vi "Modified RTS CTS.vi"() -> ()   [LabVIEW 2012]
uses:
  <vilib>/measure/maspectr.llb/FFT Power Spectrum and PSD for 1 Chan.vi
  <instrlib>/niUSRP/niUSRP Fetch Rx Data (CDB Cluster).vi
  <vilib>/addons/Modulation/Digital/General/MT Map Bits to QAM Symbols.vi
  <instrlib>/niUSRP/niUSRP Write Tx Data (CDB).vi
  <vilib>/Analysis/2dsp.llb/Inverse Complex FFT.vi
  <instrlib>/niUSRP/niUSRP Fetch Rx Data (CDB).vi
  <vilib>/Analysis/2dsp.llb/Complex FFT.vi
  <vilib>/addons/Modulation/Digital/General/MT Map QAM Symbols to Bits.vi
  <vilib>/addons/Modulation/Digital/General/MT Generate PSK System Parameters(M).vi
  <instrlib>/niUSRP/niUSRP Write Tx Data (CDB Cluster).vi
  <vilib>/Analysis/NI_AALPro.lvlib
  <vilib>/addons/Modulation/niDMT.lvlib
  <vilib>/measure/NI_MAPro.lvlib
panel:
  in  "stop 2":bool
  out "String":string
  in  "millisecond multiple":u32
  out "millisecond timer value 5":u32
  out "Enter control signal (1,2 or 3)\n1. Power\n2. Trade Off\n3. Bandwidth 2":string
  out "Symbol Rate\n[symbols/sec]":dbl=25000.0 format="%#.6p"
  in  "BPSK System Parameters 9":T1={"Samples per Symbol"=8, "symbol map"=[], "Differential PSK"=enum."disable", "PSK type"=0} caption="BPSK System Parameters" {"PSK type" items=["normal", "shifted", "offset"]; "symbol map" format="%.3f"}
  in  "BPSK System Parameters 8":T1={"Samples per Symbol"=8, "symbol map"=[], "Differential PSK"=enum."disable", "PSK type"=0} caption="BPSK System Parameters" {"PSK type" items=["normal", "shifted", "offset"]; "symbol map" format="%.3f"}
  in  "BPSK System Parameters 7":T1={"Samples per Symbol"=8, "symbol map"=[], "Differential PSK"=enum."disable", "PSK type"=0} caption="BPSK System Parameters" {"PSK type" items=["normal", "shifted", "offset"]; "symbol map" format="%.3f"}
  in  "BPSK System Parameters 6":T1={"Samples per Symbol"=8, "symbol map"=[], "Differential PSK"=enum."disable", "PSK type"=0} caption="BPSK System Parameters" {"PSK type" items=["normal", "shifted", "offset"]; "symbol map" format="%.3f"}
  in  "BPSK System Parameters 5":T1={"Samples per Symbol"=8, "symbol map"=[], "Differential PSK"=enum."disable", "PSK type"=0} caption="BPSK System Parameters" {"PSK type" items=["normal", "shifted", "offset"]; "symbol map" format="%.3f"}
  in  "BPSK System Parameters 4":T1={"Samples per Symbol"=8, "symbol map"=[], "Differential PSK"=enum."disable", "PSK type"=0} caption="BPSK System Parameters" {"PSK type" items=["normal", "shifted", "offset"]; "symbol map" format="%.3f"}
  in  "BPSK System Parameters 3":T1={"Samples per Symbol"=8, "symbol map"=[], "Differential PSK"=enum."disable", "PSK type"=0} caption="BPSK System Parameters" {"PSK type" items=["normal", "shifted", "offset"]; "symbol map" format="%.3f"}
  in  "Tab Control 3":T2(tab)
  in  "Enter control signal (1,2 or 3)\n1. Power\n2. Trade Off\n3. Bandwidth":string
  in  "Packet Parameters":T3={"Guard Bits "=30, "Sync Bits"=20, "Message Bits"=128}
  in  "Packet Pad \n[samples]":i32=200
  in  "Blank Frame \n[samples]":i32=500
  out "Number of Packets in Message":i32=46
  in  "PN sequence order\nfor Sync Bits":i32=31 caption="PN sequence order (9)"
  in  "Packet Repeat":i32=2
  in  "Pulse Shaping Filter Parameters":T4={"Alpha"=0.5, "Filter Length"=6, "TX Filter"=enum."Root Raised Cos"} caption="Pulse Shaping Filter" {"Alpha" format="%.2f"}
  in  "Tx Parameters":T5={"Tx IQ Sampling\nRate [s/sec]"=500000.0, "Tx Frequency [Hz]"=2500000000.0, "Tx Gain [dB]"=0.0, "Tx Antenna"="TX1"} {"Tx Gain [dB]" format="%#.6p"; "Tx Frequency [Hz]" format="%#.6p"; "Tx IQ Sampling\nRate [s/sec]" format="%#.6p"}
  out "Actual Tx Parameters":T5={"Tx IQ Sampling\nRate [s/sec]"=200000.0, "Tx Frequency [Hz]"=2500000000.0, "Tx Gain [dB]"=0.0, "Tx Antenna"="TX1"} {"Tx Gain [dB]" format="%#.6p"; "Tx Frequency [Hz]" format="%#.6p"; "Tx IQ Sampling\nRate [s/sec]" format="%#.6p"}
  in  "USRP IP address":refnum<k15>="192.168.10.2"
  out "error out 4":errorcluster
  in  "Queue Length":i32=10
  in  "stop":bool
  out "result":bool
  out "Constellation Graph":T6(graph)
  in  "autoscale":bool
  in  "millisecond multiple 2":u32
  out "millisecond timer value 4":u32
  out "x = y?":bool
  out "Boolean":bool
  out "Message Text 3":string="Two roads diverged in a yellow wood,\nAnd sorry I could not travel both\nAnd be one traveler, long I stood\nAnd looked down one as far as I could\nTo where it bent in the undergrowth.\n\nThen took the other, as just as fair,\nAnd having perhaps the better claim,\nBecause it was grassy and wanted wear;\nThough as for that the passing there\nHad worn them really about the same.\n\nAnd both that morning equally lay\nIn leaves no step had trodden black.\nOh, I kept the first for another day!\nYet knowing how way leads on to way,\nI doubted if I should ever come back.\n\nI shall be telling this with a sigh\nSomewhere ages and ages hence:\nTwo roads diverged in a wood, and I--\nI took the one less traveled by,\nAnd that has made all the difference.\n"
  out "M-PSK (4)":i32
  in  "Tx Parameters 3":T5={"Tx IQ Sampling\nRate [s/sec]"=500000.0, "Tx Frequency [Hz]"=2500000000.0, "Tx Gain [dB]"=0.0, "Tx Antenna"="TX1"} {"Tx Gain [dB]" format="%#.6p"; "Tx Frequency [Hz]" format="%#.6p"; "Tx IQ Sampling\nRate [s/sec]" format="%#.6p"}
  in  "Tx Parameters 2":T5={"Tx IQ Sampling\nRate [s/sec]"=500000.0, "Tx Frequency [Hz]"=2500000000.0, "Tx Gain [dB]"=0.0, "Tx Antenna"="TX1"} {"Tx Gain [dB]" format="%#.6p"; "Tx Frequency [Hz]" format="%#.6p"; "Tx IQ Sampling\nRate [s/sec]" format="%#.6p"}
  out "millisecond timer value 3":u32
  out "Magnitude":dbl[](graph)
  out "Phase":dbl[](graph)
  out "FFT {X}":dbl[](graph)
  out "theta":dbl[](graph)
  out "Unequalized Data":cdb[](graph)
  out "Equalized Data":cdb[](graph)
  out "output bit stream 2":i8[][](array[numeric])
  in  "Tab Control 2":enum32{"Parameters", "Debug", "CFO"}(tab)
  in  "Active antenna":string="RX1"
  in  "Gain":dbl=3.0 format="%#_6f"
  in  "Carrier frequency":dbl=910000000.0 format="%#_6p"
  in  "IQ rate 3":dbl=5000000.0 format="%#_6p"
  in  "Number of samples":i64=1600
  out "Coerced IQ rate":dbl=100000.0 format="%#_6p"
  out "Output bit stream":i8[](array[numeric]) caption="output bit stream"
  out "error out 2":errorcluster
  out "error out 3":errorcluster
  out "CFOest (Hz)":dbl[](array[numeric])
  out "output bit stream 3":i8[][](array[numeric])
  in  "Reference Array":dbl[](array[numeric])
  out "millisecond timer value":u32
  out "X":cdb[](array[numeric])
  out "Array out":cdb[](array[numeric])
  out "Interleaved Output":cdb[](array[numeric])
  out "Output with CP":cdb[](array[numeric])
  out "Data Size":i32
  out "Reference Symbols \n         Added":i32
  out "After Zero \n  Padding":i32
  out "After CP":i32
  out "Outgoing Constellation":cdb[](graph)=[-0.7071067811865476-0.7071067811865476i, -0.7071067811865476-0.7071067811865476i, -0.7071067811865476-0.7071067811865476i, 0.7071067811865476-0.7071067811865476i, 0.7071067811865476-0.7071067811865476i, 0.7071067811865476+0.7071067811865476i, 0.7071067811865476-0.7071067811865476i, -0.7071067811865476-0.7071067811865476i, 0.7071067811865476+0.7071067811865476i, -0.7071067811865476+0.7071067811865476i, -0.7071067811865476-0.7071067811865476i, -0.7071067811865476+0.7071067811865476i, -0.7071067811865476+0.7071067811865476i, 0.7071067811865476-0.7071067811865476i, -0.7071067811865476+0.7071067811865476i, -0.7071067811865476+0.7071067811865476i, 0.7071067811865476-0.7071067811865476i, -0.7071067811865476+0.7071067811865476i, -0.7071067811865476-0.7071067811865476i, 0.7071067811865476-0.7071067811865476i, 0.7071067811865476+0.7071067811865476i, -0.7071067811865476-0.7071067811865476i, -0.7071067811865476-0.7071067811865476i, 0.7071067811865476-0.7071067811865476i, -0.7071067811865476-0.7071067811865476i, 0.7071067811865476-0.7071067811865476i, 0.7071067811865476-0.7071067811865476i, 0.7071067811865476+0.7071067811865476i, 0.7071067811865476+0.7071067811865476i, -0.7071067811865476-0.7071067811865476i, -0.7071067811865476+0.7071067811865476i, -0.7071067811865476+0.7071067811865476i, 0.7071067811865476-0.7071067811865476i, -0.7071067811865476-0.7071067811865476i, -0.7071067811865476+0.7071067811865476i, -0.7071067811865476-0.7071067811865476i, -0.7071067811865476+0.7071067811865476i, 0.7071067811865476-0.7071067811865476i, 0.7071067811865476+0.7071067811865476i, 0.7071067811865476+0.7071067811865476i, 0.7071067811865476-0.7071067811865476i, -0.7071067811865476-0.7071067811865476i, -0.7071067811865476+0.7071067811865476i, -0.7071067811865476+0.7071067811865476i, -0.7071067811865476-0.7071067811865476i, -0.7071067811865476-0.7071067811865476i, -0.7071067811865476+0.7071067811865476i, -0.7071067811865476+0.7071067811865476i, -0.7071067811865476+0.7071067811865476i, -0.7071067811865476+0.7071067811865476i, 0.7071067811865476+0.7071067811865476i, 0.7071067811865476+0.7071067811865476i, 0.7071067811865476+0.7071067811865476i, 0.7071067811865476-0.7071067811865476i, 0.7071067811865476-0.7071067811865476i, -0.7071067811865476+0.7071067811865476i, -0.7071067811865476+0.7071067811865476i, -0.7071067811865476+0.7071067811865476i, -0.7071067811865476-0.7071067811865476i, 0.7071067811865476-0.7071067811865476i, -0.7071067811865476+0.7071067811865476i, -0.7071067811865476+0.7071067811865476i, -0.7071067811865476-0.7071067811865476i, -0.7071067811865476+0.7071067811865476i, -0.7071067811865476-0.7071067811865476i, 0.7071067811865476+0.7071067811865476i, 0.7071067811865476+0.7071067811865476i, 0.7071067811865476+0.7071067811865476i, -0.7071067811865476-0.7071067811865476i, 0.7071067811865476-0.7071067811865476i, -0.7071067811865476+0.7071067811865476i, -0.7071067811865476-0.7071067811865476i, -0.7071067811865476+0.7071067811865476i, 0.7071067811865476+0.7071067811865476i, 0.7071067811865476-0.7071067811865476i, -0.7071067811865476+0.7071067811865476i, -0.7071067811865476-0.7071067811865476i, 0.7071067811865476-0.7071067811865476i, 0.7071067811865476-0.7071067811865476i, -0.7071067811865476-0.7071067811865476i, 0.7071067811865476-0.7071067811865476i, 0.7071067811865476-0.7071067811865476i, 0.7071067811865476-0.7071067811865476i, 0.7071067811865476+0.7071067811865476i, 0.7071067811865476-0.7071067811865476i, -0.7071067811865476+0.7071067811865476i, 0.7071067811865476+0.7071067811865476i, 0.7071067811865476+0.7071067811865476i, -0.7071067811865476-0.7071067811865476i, 0.7071067811865476+0.7071067811865476i, -0.7071067811865476-0.7071067811865476i, 0.7071067811865476-0.7071067811865476i, 0.7071067811865476+0.7071067811865476i, -0.7071067811865476+0.7071067811865476i, -0.7071067811865476+0.7071067811865476i, -0.7071067811865476-0.7071067811865476i, 0.7071067811865476-0.7071067811865476i, -0.7071067811865476-0.7071067811865476i, -0.7071067811865476+0.7071067811865476i, 0.7071067811865476-0.7071067811865476i, -0.7071067811865476+0.7071067811865476i, 0.7071067811865476-0.7071067811865476i, 0.7071067811865476-0.7071067811865476i, 0.7071067811865476+0.7071067811865476i, -0.7071067811865476+0.7071067811865476i, -0.7071067811865476-0.7071067811865476i, -0.7071067811865476+0.7071067811865476i, -0.7071067811865476-0.7071067811865476i, 0.7071067811865476-0.7071067811865476i, 0.7071067811865476+0.7071067811865476i, -0.7071067811865476+0.7071067811865476i, -0.7071067811865476-0.7071067811865476i, -0.7071067811865476-0.7071067811865476i, -0.7071067811865476-0.7071067811865476i, -0.7071067811865476-0.7071067811865476i, 0.7071067811865476+0.7071067811865476i, 0.7071067811865476+0.7071067811865476i, -0.7071067811865476+0.7071067811865476i, -0.7071067811865476-0.7071067811865476i, 0.7071067811865476-0.7071067811865476i, -0.7071067811865476-0.7071067811865476i, -0.7071067811865476-0.7071067811865476i, 0.7071067811865476-0.7071067811865476i, 0.7071067811865476+0.7071067811865476i, 0.7071067811865476-0.7071067811865476i, -0.7071067811865476-0.7071067811865476i, 0.7071067811865476-0.7071067811865476i, -0.7071067811865476+0.7071067811865476i, 0.7071067811865476-0.7071067811865476i, -0.7071067811865476+0.7071067811865476i, 0.7071067811865476+0.7071067811865476i, 0.7071067811865476+0.7071067811865476i, -0.7071067811865476+0.7071067811865476i, 0.7071067811865476+0.7071067811865476i, 0.7071067811865476-0.7071067811865476i, 0.7071067811865476-0.7071067811865476i, -0.7071067811865476+0.7071067811865476i, -0.7071067811865476-0.7071067811865476i, -0.7071067811865476+0.7071067811865476i, 0.7071067811865476-0.7071067811865476i, 0.7071067811865476-0.7071067811865476i, 0.7071067811865476+0.7071067811865476i, -0.7071067811865476-0.7071067811865476i, -0.7071067811865476-0.7071067811865476i, 0.7071067811865476+0.7071067811865476i, -0.7071067811865476-0.7071067811865476i, -0.7071067811865476-0.7071067811865476i, 0.7071067811865476-0.7071067811865476i, -0.7071067811865476+0.7071067811865476i, 0.7071067811865476-0.7071067811865476i, -0.7071067811865476-0.7071067811865476i, 0.7071067811865476+0.7071067811865476i, -0.7071067811865476+0.7071067811865476i, -0.7071067811865476+0.7071067811865476i, -0.7071067811865476+0.7071067811865476i, 0.7071067811865476+0.7071067811865476i, 0.7071067811865476-0.7071067811865476i, 0.7071067811865476+0.7071067811865476i, -0.7071067811865476-0.7071067811865476i, 0.7071067811865476-0.7071067811865476i, 0.7071067811865476+0.7071067811865476i, -0.7071067811865476-0.7071067811865476i, -0.7071067811865476+0.7071067811865476i, 0.7071067811865476-0.7071067811865476i, 0.7071067811865476-0.7071067811865476i, 0.7071067811865476-0.7071067811865476i, -0.7071067811865476-0.7071067811865476i, 0.7071067811865476-0.7071067811865476i, 0.7071067811865476+0.7071067811865476i, 0.7071067811865476-0.7071067811865476i, -0.7071067811865476+0.7071067811865476i, 0.7071067811865476-0.7071067811865476i, 0.7071067811865476+0.7071067811865476i, 0.7071067811865476-0.7071067811865476i, 0.7071067811865476+0.7071067811865476i, 0.7071067811865476-0.7071067811865476i, 0.7071067811865476+0.7071067811865476i, 0.7071067811865476+0.7071067811865476i, 0.7071067811865476+0.7071067811865476i, -0.7071067811865476+0.7071067811865476i, 0.7071067811865476+0.7071067811865476i, 0.7071067811865476+0.7071067811865476i, 0.7071067811865476-0.7071067811865476i, 0.7071067811865476+0.7071067811865476i, -0.7071067811865476-0.7071067811865476i, 0.7071067811865476+0.7071067811865476i, 0.7071067811865476+0.7071067811865476i, 0.7071067811865476-0.7071067811865476i, -0.7071067811865476+0.7071067811865476i, -0.7071067811865476-0.7071067811865476i, 0.7071067811865476+0.7071067811865476i, 0.7071067811865476-0.7071067811865476i, 0.7071067811865476-0.7071067811865476i, 0.7071067811865476-0.7071067811865476i, -0.7071067811865476-0.7071067811865476i, 0.7071067811865476+0.7071067811865476i, 0.7071067811865476+0.7071067811865476i, -0.7071067811865476-0.7071067811865476i, -0.7071067811865476+0.7071067811865476i, -0.7071067811865476-0.7071067811865476i, 0.7071067811865476-0.7071067811865476i, 0.7071067811865476-0.7071067811865476i, -0.7071067811865476+0.7071067811865476i, 0.7071067811865476-0.7071067811865476i, -0.7071067811865476-0.7071067811865476i, 0.7071067811865476-0.7071067811865476i, -0.7071067811865476+0.7071067811865476i, 0.7071067811865476+0.7071067811865476i, -0.7071067811865476+0.7071067811865476i, -0.7071067811865476+0.7071067811865476i, 0.7071067811865476+0.7071067811865476i, 0.7071067811865476+0.7071067811865476i, 0.7071067811865476-0.7071067811865476i, 0.7071067811865476-0.7071067811865476i, -0.7071067811865476-0.7071067811865476i, -0.7071067811865476+0.7071067811865476i, 0.7071067811865476+0.7071067811865476i, -0.7071067811865476-0.7071067811865476i, -0.7071067811865476-0.7071067811865476i, -0.7071067811865476-0.7071067811865476i, -0.7071067811865476+0.7071067811865476i, 0.7071067811865476-0.7071067811865476i, -0.7071067811865476+0.7071067811865476i, 0.7071067811865476+0.7071067811865476i, 0.7071067811865476-0.7071067811865476i, -0.7071067811865476+0.7071067811865476i, -0.7071067811865476+0.7071067811865476i, 0.7071067811865476-0.7071067811865476i, -0.7071067811865476-0.7071067811865476i, -0.7071067811865476-0.7071067811865476i, -0.7071067811865476-0.7071067811865476i, 0.7071067811865476+0.7071067811865476i, 0.7071067811865476-0.7071067811865476i, -0.7071067811865476+0.7071067811865476i, 0.7071067811865476-0.7071067811865476i, 0.7071067811865476-0.7071067811865476i, 0.7071067811865476-0.7071067811865476i, -0.7071067811865476+0.7071067811865476i, 0.7071067811865476-0.7071067811865476i, -0.7071067811865476+0.7071067811865476i, 0.7071067811865476-0.7071067811865476i, 0.7071067811865476+0.7071067811865476i, 0.7071067811865476+0.7071067811865476i, 0.7071067811865476+0.7071067811865476i, -0.7071067811865476-0.7071067811865476i, 0.7071067811865476+0.7071067811865476i, -0.7071067811865476+0.7071067811865476i, 0.7071067811865476-0.7071067811865476i, -0.7071067811865476+0.7071067811865476i, -0.7071067811865476+0.7071067811865476i, 0.7071067811865476+0.7071067811865476i, -0.7071067811865476+0.7071067811865476i, 0.7071067811865476-0.7071067811865476i, 0.7071067811865476-0.7071067811865476i, -0.7071067811865476+0.7071067811865476i, -0.7071067811865476+0.7071067811865476i, -0.7071067811865476-0.7071067811865476i, -0.7071067811865476-0.7071067811865476i, -0.7071067811865476-0.7071067811865476i, -0.7071067811865476+0.7071067811865476i, 0.7071067811865476+0.7071067811865476i, -0.7071067811865476+0.7071067811865476i, -0.7071067811865476+0.7071067811865476i, 0.7071067811865476-0.7071067811865476i, 0.7071067811865476+0.7071067811865476i, -0.7071067811865476-0.7071067811865476i, 0.7071067811865476-0.7071067811865476i, 0.7071067811865476-0.7071067811865476i, -0.7071067811865476-0.7071067811865476i, 0.7071067811865476+0.7071067811865476i, 0.7071067811865476-0.7071067811865476i, -0.7071067811865476-0.7071067811865476i, 0.7071067811865476+0.7071067811865476i, -0.7071067811865476-0.7071067811865476i, -0.7071067811865476-0.7071067811865476i, 0.7071067811865476+0.7071067811865476i, -0.7071067811865476+0.7071067811865476i, -0.7071067811865476-0.7071067811865476i, -0.7071067811865476-0.7071067811865476i, -0.7071067811865476+0.7071067811865476i, -0.7071067811865476-0.7071067811865476i, -0.7071067811865476+0.7071067811865476i, 0.7071067811865476+0.7071067811865476i, 0.7071067811865476+0.7071067811865476i, -0.7071067811865476+0.7071067811865476i, 0.7071067811865476-0.7071067811865476i, 0.7071067811865476-0.7071067811865476i, -0.7071067811865476-0.7071067811865476i, -0.7071067811865476+0.7071067811865476i, 0.7071067811865476-0.7071067811865476i, -0.7071067811865476-0.7071067811865476i, 0.7071067811865476-0.7071067811865476i, -0.7071067811865476-0.7071067811865476i, 0.7071067811865476+0.7071067811865476i, 0.7071067811865476+0.7071067811865476i, -0.7071067811865476+0.7071067811865476i, -0.7071067811865476+0.7071067811865476i, 0.7071067811865476-0.7071067811865476i, 0.7071067811865476-0.7071067811865476i, -0.7071067811865476-0.7071067811865476i, -0.7071067811865476-0.7071067811865476i, 0.7071067811865476-0.7071067811865476i, 0.7071067811865476-0.7071067811865476i, 0.7071067811865476-0.7071067811865476i, 0.7071067811865476-0.7071067811865476i, 0.7071067811865476-0.7071067811865476i, 0.7071067811865476+0.7071067811865476i, 0.7071067811865476+0.7071067811865476i, -0.7071067811865476+0.7071067811865476i, -0.7071067811865476+0.7071067811865476i, 0.7071067811865476+0.7071067811865476i, 0.7071067811865476-0.7071067811865476i, 0.7071067811865476-0.7071067811865476i, -0.7071067811865476-0.7071067811865476i, -0.7071067811865476-0.7071067811865476i, 0.7071067811865476+0.7071067811865476i, 0.7071067811865476-0.7071067811865476i, -0.7071067811865476-0.7071067811865476i, 0.7071067811865476-0.7071067811865476i, -0.7071067811865476-0.7071067811865476i, 0.7071067811865476-0.7071067811865476i, 0.7071067811865476+0.7071067811865476i, 0.7071067811865476+0.7071067811865476i, -0.7071067811865476+0.7071067811865476i, -0.7071067811865476-0.7071067811865476i, 0.7071067811865476+0.7071067811865476i, -0.7071067811865476-0.7071067811865476i, 0.7071067811865476-0.7071067811865476i, 0.7071067811865476-0.7071067811865476i, -0.7071067811865476+0.7071067811865476i, 0.7071067811865476+0.7071067811865476i, -0.7071067811865476-0.7071067811865476i, -0.7071067811865476-0.7071067811865476i, -0.7071067811865476+0.7071067811865476i, -0.7071067811865476+0.7071067811865476i, -0.7071067811865476-0.7071067811865476i, -0.7071067811865476+0.7071067811865476i, -0.7071067811865476+0.7071067811865476i, 0.7071067811865476+0.7071067811865476i, -0.7071067811865476+0.7071067811865476i, 0.7071067811865476+0.7071067811865476i, 0.7071067811865476-0.7071067811865476i, 0.7071067811865476+0.7071067811865476i, -0.7071067811865476+0.7071067811865476i, 0.7071067811865476-0.7071067811865476i, -0.7071067811865476+0.7071067811865476i, -0.7071067811865476-0.7071067811865476i, 0.7071067811865476+0.7071067811865476i, 0.7071067811865476+0.7071067811865476i, 0.7071067811865476-0.7071067811865476i, -0.7071067811865476-0.7071067811865476i, -0.7071067811865476-0.7071067811865476i, -0.7071067811865476+0.7071067811865476i, 0.7071067811865476-0.7071067811865476i, -0.7071067811865476-0.7071067811865476i, 0.7071067811865476+0.7071067811865476i, -0.7071067811865476-0.7071067811865476i, -0.7071067811865476+0.7071067811865476i, 0.7071067811865476+0.7071067811865476i, 0.7071067811865476+0.7071067811865476i, -0.7071067811865476-0.7071067811865476i, 0.7071067811865476-0.7071067811865476i, -0.7071067811865476-0.7071067811865476i, -0.7071067811865476-0.7071067811865476i, 0.7071067811865476+0.7071067811865476i, 0.7071067811865476+0.7071067811865476i, -0.7071067811865476-0.7071067811865476i, -0.7071067811865476-0.7071067811865476i, -0.7071067811865476-0.7071067811865476i, -0.7071067811865476-0.7071067811865476i, 0.7071067811865476-0.7071067811865476i, 0.7071067811865476+0.7071067811865476i, 0.7071067811865476+0.7071067811865476i, -0.7071067811865476-0.7071067811865476i, -0.7071067811865476-0.7071067811865476i, -0.7071067811865476+0.7071067811865476i, -0.7071067811865476-0.7071067811865476i, -0.7071067811865476-0.7071067811865476i, 0.7071067811865476+0.7071067811865476i, -0.7071067811865476+0.7071067811865476i, -0.7071067811865476+0.7071067811865476i, -0.7071067811865476-0.7071067811865476i, 0.7071067811865476+0.7071067811865476i, -0.7071067811865476-0.7071067811865476i, 0.7071067811865476+0.7071067811865476i, 0.7071067811865476-0.7071067811865476i, 0.7071067811865476+0.7071067811865476i, 0.7071067811865476+0.7071067811865476i, 0.7071067811865476-0.7071067811865476i, -0.7071067811865476+0.7071067811865476i, -0.7071067811865476+0.7071067811865476i, 0.7071067811865476+0.7071067811865476i, -0.7071067811865476-0.7071067811865476i, 0.7071067811865476-0.7071067811865476i, -0.7071067811865476-0.7071067811865476i, -0.7071067811865476+0.7071067811865476i, 0.7071067811865476+0.7071067811865476i, -0.7071067811865476+0.7071067811865476i, -0.7071067811865476-0.7071067811865476i, 0.7071067811865476-0.7071067811865476i, -0.7071067811865476+0.7071067811865476i, -0.7071067811865476-0.7071067811865476i, -0.7071067811865476-0.7071067811865476i, 0.7071067811865476+0.7071067811865476i, -0.7071067811865476-0.7071067811865476i, -0.7071067811865476+0.7071067811865476i, 0.7071067811865476-0.7071067811865476i, 0.7071067811865476+0.7071067811865476i, 0.7071067811865476-0.7071067811865476i, 0.7071067811865476-0.7071067811865476i, 0.7071067811865476-0.7071067811865476i, -0.7071067811865476+0.7071067811865476i, 0.7071067811865476+0.7071067811865476i, -0.7071067811865476+0.7071067811865476i, -0.7071067811865476-0.7071067811865476i, 0.7071067811865476+0.7071067811865476i, -0.7071067811865476+0.7071067811865476i, 0.7071067811865476-0.7071067811865476i, -0.7071067811865476-0.7071067811865476i, -0.7071067811865476+0.7071067811865476i, -0.7071067811865476+0.7071067811865476i, -0.7071067811865476+0.7071067811865476i, -0.7071067811865476-0.7071067811865476i, 0.7071067811865476+0.7071067811865476i, -0.7071067811865476+0.7071067811865476i, 0.7071067811865476+0.7071067811865476i, -0.7071067811865476-0.7071067811865476i, 0.7071067811865476+0.7071067811865476i, -0.7071067811865476+0.7071067811865476i, 0.7071067811865476+0.7071067811865476i, -0.7071067811865476+0.7071067811865476i, 0.7071067811865476+0.7071067811865476i, 0.7071067811865476+0.7071067811865476i, 0.7071067811865476+0.7071067811865476i, 0.7071067811865476+0.7071067811865476i, 0.7071067811865476-0.7071067811865476i, 0.7071067811865476+0.7071067811865476i, -0.7071067811865476+0.7071067811865476i, 0.7071067811865476+0.7071067811865476i, -0.7071067811865476+0.7071067811865476i, 0.7071067811865476-0.7071067811865476i, 0.7071067811865476+0.7071067811865476i, -0.7071067811865476+0.7071067811865476i, 0.7071067811865476+0.7071067811865476i, -0.7071067811865476-0.7071067811865476i, 0.7071067811865476-0.7071067811865476i, -0.7071067811865476+0.7071067811865476i, -0.7071067811865476+0.7071067811865476i, -0.7071067811865476+0.7071067811865476i, -0.7071067811865476+0.7071067811865476i, 0.7071067811865476-0.7071067811865476i, 0.7071067811865476+0.7071067811865476i, -0.7071067811865476+0.7071067811865476i, 0.7071067811865476-0.7071067811865476i, -0.7071067811865476-0.7071067811865476i, -0.7071067811865476-0.7071067811865476i, -0.7071067811865476+0.7071067811865476i, 0.7071067811865476+0.7071067811865476i, -0.7071067811865476-0.7071067811865476i, -0.7071067811865476+0.7071067811865476i, -0.7071067811865476-0.7071067811865476i, 0.7071067811865476+0.7071067811865476i, 0.7071067811865476-0.7071067811865476i, 0.7071067811865476+0.7071067811865476i, 0.7071067811865476-0.7071067811865476i, 0.7071067811865476-0.7071067811865476i, 0.7071067811865476+0.7071067811865476i, -0.7071067811865476+0.7071067811865476i, -0.7071067811865476+0.7071067811865476i, -0.7071067811865476+0.7071067811865476i, 0.7071067811865476-0.7071067811865476i, 0.7071067811865476-0.7071067811865476i, -0.7071067811865476+0.7071067811865476i, -0.7071067811865476-0.7071067811865476i, -0.7071067811865476-0.7071067811865476i, 0.7071067811865476-0.7071067811865476i, -0.7071067811865476-0.7071067811865476i, 0.7071067811865476+0.7071067811865476i, 0.7071067811865476-0.7071067811865476i, -0.7071067811865476+0.7071067811865476i, 0.7071067811865476+0.7071067811865476i, 0.7071067811865476-0.7071067811865476i, -0.7071067811865476-0.7071067811865476i, -0.7071067811865476+0.7071067811865476i, -0.7071067811865476-0.7071067811865476i, -0.7071067811865476-0.7071067811865476i, 0.7071067811865476-0.7071067811865476i, -0.7071067811865476+0.7071067811865476i, 0.7071067811865476+0.7071067811865476i, -0.7071067811865476-0.7071067811865476i, -0.7071067811865476+0.7071067811865476i, -0.7071067811865476+0.7071067811865476i, 0.7071067811865476+0.7071067811865476i, -0.7071067811865476-0.7071067811865476i, 0.7071067811865476+0.7071067811865476i, -0.7071067811865476-0.7071067811865476i, 0.7071067811865476+0.7071067811865476i, 0.7071067811865476+0.7071067811865476i, 0.7071067811865476+0.7071067811865476i, -0.7071067811865476+0.7071067811865476i, 0.7071067811865476-0.7071067811865476i, 0.7071067811865476+0.7071067811865476i, -0.7071067811865476-0.7071067811865476i, 0.7071067811865476+0.7071067811865476i, 0.7071067811865476-0.7071067811865476i, 0.7071067811865476-0.7071067811865476i, 0.7071067811865476+0.7071067811865476i, -0.7071067811865476-0.7071067811865476i, -0.7071067811865476+0.7071067811865476i, 0.7071067811865476+0.7071067811865476i, 0.7071067811865476-0.7071067811865476i, -0.7071067811865476-0.7071067811865476i, -0.7071067811865476-0.7071067811865476i, -0.7071067811865476-0.7071067811865476i, 0.7071067811865476-0.7071067811865476i, 0.7071067811865476-0.7071067811865476i, 0.7071067811865476+0.7071067811865476i, 0.7071067811865476-0.7071067811865476i, -0.7071067811865476-0.7071067811865476i, 0.7071067811865476+0.7071067811865476i, -0.7071067811865476+0.7071067811865476i, -0.7071067811865476-0.7071067811865476i, -0.7071067811865476+0.7071067811865476i, -0.7071067811865476+0.7071067811865476i, 0.7071067811865476-0.7071067811865476i, -0.7071067811865476+0.7071067811865476i, -0.7071067811865476+0.7071067811865476i, 0.7071067811865476-0.7071067811865476i, -0.7071067811865476+0.7071067811865476i, -0.7071067811865476-0.7071067811865476i, 0.7071067811865476-0.7071067811865476i, 0.7071067811865476+0.7071067811865476i, -0.7071067811865476-0.7071067811865476i, -0.7071067811865476-0.7071067811865476i, 0.7071067811865476-0.7071067811865476i, -0.7071067811865476-0.7071067811865476i, 0.7071067811865476-0.7071067811865476i, 0.7071067811865476-0.7071067811865476i, 0.7071067811865476+0.7071067811865476i, 0.7071067811865476+0.7071067811865476i, -0.7071067811865476-0.7071067811865476i, -0.7071067811865476+0.7071067811865476i, -0.7071067811865476+0.7071067811865476i, 0.7071067811865476-0.7071067811865476i, -0.7071067811865476-0.7071067811865476i, -0.7071067811865476+0.7071067811865476i, -0.7071067811865476-0.7071067811865476i, -0.7071067811865476+0.7071067811865476i, 0.7071067811865476-0.7071067811865476i, 0.7071067811865476+0.7071067811865476i, 0.7071067811865476+0.7071067811865476i, 0.7071067811865476-0.7071067811865476i, -0.7071067811865476-0.7071067811865476i, -0.7071067811865476+0.7071067811865476i, -0.7071067811865476+0.7071067811865476i, -0.7071067811865476-0.7071067811865476i, -0.7071067811865476-0.7071067811865476i, -0.7071067811865476+0.7071067811865476i, -0.7071067811865476+0.7071067811865476i, -0.7071067811865476+0.7071067811865476i, -0.7071067811865476+0.7071067811865476i, 0.7071067811865476+0.7071067811865476i, 0.7071067811865476+0.7071067811865476i, 0.7071067811865476+0.7071067811865476i, 0.7071067811865476-0.7071067811865476i, 0.7071067811865476-0.7071067811865476i, -0.7071067811865476+0.7071067811865476i, -0.7071067811865476+0.7071067811865476i, -0.7071067811865476+0.7071067811865476i, -0.7071067811865476-0.7071067811865476i, 0.7071067811865476-0.7071067811865476i, -0.7071067811865476+0.7071067811865476i, -0.7071067811865476+0.7071067811865476i, -0.7071067811865476-0.7071067811865476i, -0.7071067811865476+0.7071067811865476i, -0.7071067811865476-0.7071067811865476i, 0.7071067811865476+0.7071067811865476i, 0.7071067811865476+0.7071067811865476i, 0.7071067811865476+0.7071067811865476i, -0.7071067811865476-0.7071067811865476i, 0.7071067811865476-0.7071067811865476i, -0.7071067811865476+0.7071067811865476i, -0.7071067811865476-0.7071067811865476i, -0.7071067811865476+0.7071067811865476i, 0.7071067811865476+0.7071067811865476i, 0.7071067811865476-0.7071067811865476i, -0.7071067811865476+0.7071067811865476i, -0.7071067811865476-0.7071067811865476i, 0.7071067811865476-0.7071067811865476i, 0.7071067811865476-0.7071067811865476i, -0.7071067811865476-0.7071067811865476i, 0.7071067811865476-0.7071067811865476i, 0.7071067811865476-0.7071067811865476i, 0.7071067811865476-0.7071067811865476i, 0.7071067811865476+0.7071067811865476i, 0.7071067811865476-0.7071067811865476i, -0.7071067811865476+0.7071067811865476i, 0.7071067811865476+0.7071067811865476i, 0.7071067811865476+0.7071067811865476i, -0.7071067811865476-0.7071067811865476i, 0.7071067811865476+0.7071067811865476i, -0.7071067811865476-0.7071067811865476i, 0.7071067811865476-0.7071067811865476i, 0.7071067811865476+0.7071067811865476i, -0.7071067811865476+0.7071067811865476i, -0.7071067811865476+0.7071067811865476i, -0.7071067811865476-0.7071067811865476i, 0.7071067811865476-0.7071067811865476i, -0.7071067811865476-0.7071067811865476i, -0.7071067811865476+0.7071067811865476i, 0.7071067811865476-0.7071067811865476i, -0.7071067811865476+0.7071067811865476i, 0.7071067811865476-0.7071067811865476i, 0.7071067811865476-0.7071067811865476i, 0.7071067811865476+0.7071067811865476i, -0.7071067811865476+0.7071067811865476i, -0.7071067811865476-0.7071067811865476i, -0.7071067811865476+0.7071067811865476i, -0.7071067811865476-0.7071067811865476i, 0.7071067811865476-0.7071067811865476i, 0.7071067811865476+0.7071067811865476i, -0.7071067811865476+0.7071067811865476i, -0.7071067811865476-0.7071067811865476i, -0.7071067811865476-0.7071067811865476i, -0.7071067811865476-0.7071067811865476i, -0.7071067811865476-0.7071067811865476i, 0.7071067811865476+0.7071067811865476i, 0.7071067811865476+0.7071067811865476i, -0.7071067811865476+0.7071067811865476i, -0.7071067811865476-0.7071067811865476i, 0.7071067811865476-0.7071067811865476i, -0.7071067811865476-0.7071067811865476i, -0.7071067811865476-0.7071067811865476i, 0.7071067811865476-0.7071067811865476i, 0.7071067811865476+0.7071067811865476i, 0.7071067811865476-0.7071067811865476i, -0.7071067811865476-0.7071067811865476i, 0.7071067811865476-0.7071067811865476i, -0.7071067811865476+0.7071067811865476i, 0.7071067811865476-0.7071067811865476i, -0.7071067811865476+0.7071067811865476i, 0.7071067811865476+0.7071067811865476i, 0.7071067811865476+0.7071067811865476i, -0.7071067811865476+0.7071067811865476i, 0.7071067811865476+0.7071067811865476i, 0.7071067811865476-0.7071067811865476i, 0.7071067811865476-0.7071067811865476i, -0.7071067811865476+0.7071067811865476i, -0.7071067811865476-0.7071067811865476i, -0.7071067811865476+0.7071067811865476i, 0.7071067811865476-0.7071067811865476i, 0.7071067811865476-0.7071067811865476i, 0.7071067811865476+0.7071067811865476i, -0.7071067811865476-0.7071067811865476i, -0.7071067811865476-0.7071067811865476i, 0.7071067811865476+0.7071067811865476i, -0.7071067811865476-0.7071067811865476i, -0.7071067811865476-0.7071067811865476i, 0.7071067811865476-0.7071067811865476i, -0.7071067811865476+0.7071067811865476i, 0.7071067811865476-0.7071067811865476i, -0.7071067811865476-0.7071067811865476i, 0.7071067811865476+0.7071067811865476i, -0.7071067811865476+0.7071067811865476i, -0.7071067811865476+0.7071067811865476i, -0.7071067811865476+0.7071067811865476i, 0.7071067811865476+0.7071067811865476i, 0.7071067811865476-0.7071067811865476i, 0.7071067811865476+0.7071067811865476i, -0.7071067811865476-0.7071067811865476i, 0.7071067811865476-0.7071067811865476i, 0.7071067811865476+0.7071067811865476i, -0.7071067811865476-0.7071067811865476i, -0.7071067811865476+0.7071067811865476i, 0.7071067811865476-0.7071067811865476i, 0.7071067811865476-0.7071067811865476i, 0.7071067811865476-0.7071067811865476i, -0.7071067811865476-0.7071067811865476i, 0.7071067811865476-0.7071067811865476i, 0.7071067811865476+0.7071067811865476i, 0.7071067811865476-0.7071067811865476i, -0.7071067811865476+0.7071067811865476i, 0.7071067811865476-0.7071067811865476i, 0.7071067811865476+0.7071067811865476i, 0.7071067811865476-0.7071067811865476i, 0.7071067811865476+0.7071067811865476i, 0.7071067811865476-0.7071067811865476i, 0.7071067811865476+0.7071067811865476i, 0.7071067811865476+0.7071067811865476i, 0.7071067811865476+0.7071067811865476i, -0.7071067811865476+0.7071067811865476i, 0.7071067811865476+0.7071067811865476i, 0.7071067811865476+0.7071067811865476i, 0.7071067811865476-0.7071067811865476i, 0.7071067811865476+0.7071067811865476i, -0.7071067811865476-0.7071067811865476i, 0.7071067811865476+0.7071067811865476i, 0.7071067811865476+0.7071067811865476i, 0.7071067811865476-0.7071067811865476i, -0.7071067811865476+0.7071067811865476i, -0.7071067811865476-0.7071067811865476i, 0.7071067811865476+0.7071067811865476i, 0.7071067811865476-0.7071067811865476i, 0.7071067811865476-0.7071067811865476i, 0.7071067811865476-0.7071067811865476i, -0.7071067811865476-0.7071067811865476i, 0.7071067811865476+0.7071067811865476i, 0.7071067811865476+0.7071067811865476i, -0.7071067811865476-0.7071067811865476i, -0.7071067811865476+0.7071067811865476i, -0.7071067811865476-0.7071067811865476i, 0.7071067811865476-0.7071067811865476i, 0.7071067811865476-0.7071067811865476i, -0.7071067811865476+0.7071067811865476i, 0.7071067811865476-0.7071067811865476i, -0.7071067811865476-0.7071067811865476i, 0.7071067811865476-0.7071067811865476i, -0.7071067811865476+0.7071067811865476i, 0.7071067811865476+0.7071067811865476i, -0.7071067811865476+0.7071067811865476i, -0.7071067811865476+0.7071067811865476i, 0.7071067811865476+0.7071067811865476i, 0.7071067811865476+0.7071067811865476i, 0.7071067811865476-0.7071067811865476i, 0.7071067811865476-0.7071067811865476i, -0.7071067811865476-0.7071067811865476i, -0.7071067811865476+0.7071067811865476i, 0.7071067811865476+0.7071067811865476i, -0.7071067811865476-0.7071067811865476i, -0.7071067811865476-0.7071067811865476i, -0.7071067811865476-0.7071067811865476i, -0.7071067811865476+0.7071067811865476i, 0.7071067811865476-0.7071067811865476i, -0.7071067811865476+0.7071067811865476i, 0.7071067811865476+0.7071067811865476i, 0.7071067811865476-0.7071067811865476i, -0.7071067811865476+0.7071067811865476i, -0.7071067811865476+0.7071067811865476i, 0.7071067811865476-0.7071067811865476i, -0.7071067811865476-0.7071067811865476i, -0.7071067811865476-0.7071067811865476i, -0.7071067811865476-0.7071067811865476i, 0.7071067811865476+0.7071067811865476i, 0.7071067811865476-0.7071067811865476i, -0.7071067811865476+0.7071067811865476i, 0.7071067811865476-0.7071067811865476i, 0.7071067811865476-0.7071067811865476i, 0.7071067811865476-0.7071067811865476i, -0.7071067811865476+0.7071067811865476i, 0.7071067811865476-0.7071067811865476i, -0.7071067811865476+0.7071067811865476i, 0.7071067811865476-0.7071067811865476i, 0.7071067811865476+0.7071067811865476i, 0.7071067811865476+0.7071067811865476i, 0.7071067811865476+0.7071067811865476i, -0.7071067811865476-0.7071067811865476i, 0.7071067811865476+0.7071067811865476i, -0.7071067811865476+0.7071067811865476i, 0.7071067811865476-0.7071067811865476i, -0.7071067811865476+0.7071067811865476i, -0.7071067811865476+0.7071067811865476i, 0.7071067811865476+0.7071067811865476i, -0.7071067811865476+0.7071067811865476i, 0.7071067811865476-0.7071067811865476i, 0.7071067811865476-0.7071067811865476i, -0.7071067811865476+0.7071067811865476i, -0.7071067811865476+0.7071067811865476i, -0.7071067811865476-0.7071067811865476i, -0.7071067811865476-0.7071067811865476i, -0.7071067811865476-0.7071067811865476i, -0.7071067811865476+0.7071067811865476i, 0.7071067811865476+0.7071067811865476i, -0.7071067811865476+0.7071067811865476i, -0.7071067811865476+0.7071067811865476i, 0.7071067811865476-0.7071067811865476i, 0.7071067811865476+0.7071067811865476i, -0.7071067811865476-0.7071067811865476i, 0.7071067811865476-0.7071067811865476i, 0.7071067811865476-0.7071067811865476i, -0.7071067811865476-0.7071067811865476i, 0.7071067811865476+0.7071067811865476i, 0.7071067811865476-0.7071067811865476i, -0.7071067811865476-0.7071067811865476i, 0.7071067811865476+0.7071067811865476i, -0.7071067811865476-0.7071067811865476i, -0.7071067811865476-0.7071067811865476i, 0.7071067811865476+0.7071067811865476i, -0.7071067811865476+0.7071067811865476i, -0.7071067811865476-0.7071067811865476i, -0.7071067811865476-0.7071067811865476i, -0.7071067811865476+0.7071067811865476i, -0.7071067811865476-0.7071067811865476i, -0.7071067811865476+0.7071067811865476i, 0.7071067811865476+0.7071067811865476i, 0.7071067811865476+0.7071067811865476i, -0.7071067811865476+0.7071067811865476i, 0.7071067811865476-0.7071067811865476i, 0.7071067811865476-0.7071067811865476i, -0.7071067811865476-0.7071067811865476i, -0.7071067811865476+0.7071067811865476i, 0.7071067811865476-0.7071067811865476i, -0.7071067811865476-0.7071067811865476i, 0.7071067811865476-0.7071067811865476i, -0.7071067811865476-0.7071067811865476i, 0.7071067811865476+0.7071067811865476i, 0.7071067811865476+0.7071067811865476i, -0.7071067811865476+0.7071067811865476i, -0.7071067811865476+0.7071067811865476i, 0.7071067811865476-0.7071067811865476i, 0.7071067811865476-0.7071067811865476i, -0.7071067811865476-0.7071067811865476i, -0.7071067811865476-0.7071067811865476i, 0.7071067811865476-0.7071067811865476i, 0.7071067811865476-0.7071067811865476i, 0.7071067811865476-0.7071067811865476i, 0.7071067811865476-0.7071067811865476i, 0.7071067811865476-0.7071067811865476i, 0.7071067811865476+0.7071067811865476i, 0.7071067811865476+0.7071067811865476i, -0.7071067811865476+0.7071067811865476i, -0.7071067811865476+0.7071067811865476i, 0.7071067811865476+0.7071067811865476i, 0.7071067811865476-0.7071067811865476i, 0.7071067811865476-0.7071067811865476i, -0.7071067811865476-0.7071067811865476i, -0.7071067811865476-0.7071067811865476i, 0.7071067811865476+0.7071067811865476i, 0.7071067811865476-0.7071067811865476i, -0.7071067811865476-0.7071067811865476i, 0.7071067811865476-0.7071067811865476i, -0.7071067811865476-0.7071067811865476i, 0.7071067811865476-0.7071067811865476i, 0.7071067811865476+0.7071067811865476i, 0.7071067811865476+0.7071067811865476i, -0.7071067811865476+0.7071067811865476i, -0.7071067811865476-0.7071067811865476i, 0.7071067811865476+0.7071067811865476i, -0.7071067811865476-0.7071067811865476i, 0.7071067811865476-0.7071067811865476i, 0.7071067811865476-0.7071067811865476i, -0.7071067811865476+0.7071067811865476i, 0.7071067811865476+0.7071067811865476i, -0.7071067811865476-0.7071067811865476i, -0.7071067811865476-0.7071067811865476i, -0.7071067811865476+0.7071067811865476i, -0.7071067811865476+0.7071067811865476i, -0.7071067811865476-0.7071067811865476i, -0.7071067811865476+0.7071067811865476i, -0.7071067811865476+0.7071067811865476i, 0.7071067811865476+0.7071067811865476i, -0.7071067811865476+0.7071067811865476i, 0.7071067811865476+0.7071067811865476i, 0.7071067811865476-0.7071067811865476i, 0.7071067811865476+0.7071067811865476i, -0.7071067811865476+0.7071067811865476i, 0.7071067811865476-0.7071067811865476i, -0.7071067811865476+0.7071067811865476i, -0.7071067811865476-0.7071067811865476i, 0.7071067811865476+0.7071067811865476i, 0.7071067811865476+0.7071067811865476i, 0.7071067811865476-0.7071067811865476i, -0.7071067811865476-0.7071067811865476i, -0.7071067811865476-0.7071067811865476i, -0.7071067811865476+0.7071067811865476i, 0.7071067811865476-0.7071067811865476i, -0.7071067811865476-0.7071067811865476i, 0.7071067811865476+0.7071067811865476i, -0.7071067811865476-0.7071067811865476i, -0.7071067811865476+0.7071067811865476i, 0.7071067811865476+0.7071067811865476i, 0.7071067811865476+0.7071067811865476i, -0.7071067811865476-0.7071067811865476i, 0.7071067811865476-0.7071067811865476i, -0.7071067811865476-0.7071067811865476i, -0.7071067811865476-0.7071067811865476i, 0.7071067811865476+0.7071067811865476i, 0.7071067811865476+0.7071067811865476i, -0.7071067811865476-0.7071067811865476i, -0.7071067811865476-0.7071067811865476i, -0.7071067811865476-0.7071067811865476i, -0.7071067811865476-0.7071067811865476i, 0.7071067811865476-0.7071067811865476i, 0.7071067811865476+0.7071067811865476i, 0.7071067811865476+0.7071067811865476i, -0.7071067811865476-0.7071067811865476i, -0.7071067811865476-0.7071067811865476i, -0.7071067811865476+0.7071067811865476i, -0.7071067811865476-0.7071067811865476i, -0.7071067811865476-0.7071067811865476i, 0.7071067811865476+0.7071067811865476i, -0.7071067811865476+0.7071067811865476i, -0.7071067811865476+0.7071067811865476i, -0.7071067811865476-0.7071067811865476i, 0.7071067811865476+0.7071067811865476i, -0.7071067811865476-0.7071067811865476i, 0.7071067811865476+0.7071067811865476i, 0.7071067811865476-0.7071067811865476i, 0.7071067811865476+0.7071067811865476i, 0.7071067811865476+0.7071067811865476i, 0.7071067811865476-0.7071067811865476i, -0.7071067811865476+0.7071067811865476i, -0.7071067811865476+0.7071067811865476i, 0.7071067811865476+0.7071067811865476i, -0.7071067811865476-0.7071067811865476i, 0.7071067811865476-0.7071067811865476i, -0.7071067811865476-0.7071067811865476i, -0.7071067811865476+0.7071067811865476i, 0.7071067811865476+0.7071067811865476i, -0.7071067811865476+0.7071067811865476i, -0.7071067811865476-0.7071067811865476i, 0.7071067811865476-0.7071067811865476i, -0.7071067811865476+0.7071067811865476i, -0.7071067811865476-0.7071067811865476i, -0.7071067811865476-0.7071067811865476i, 0.7071067811865476+0.7071067811865476i, -0.7071067811865476-0.7071067811865476i, -0.7071067811865476+0.7071067811865476i, 0.7071067811865476-0.7071067811865476i, 0.7071067811865476+0.7071067811865476i, 0.7071067811865476-0.7071067811865476i, 0.7071067811865476-0.7071067811865476i, 0.7071067811865476-0.7071067811865476i, -0.7071067811865476+0.7071067811865476i, 0.7071067811865476+0.7071067811865476i, -0.7071067811865476+0.7071067811865476i, -0.7071067811865476-0.7071067811865476i, 0.7071067811865476+0.7071067811865476i, -0.7071067811865476+0.7071067811865476i, 0.7071067811865476-0.7071067811865476i, -0.7071067811865476-0.7071067811865476i, -0.7071067811865476+0.7071067811865476i, -0.7071067811865476+0.7071067811865476i, -0.7071067811865476+0.7071067811865476i, -0.7071067811865476-0.7071067811865476i, 0.7071067811865476+0.7071067811865476i, -0.7071067811865476+0.7071067811865476i, 0.7071067811865476+0.7071067811865476i, -0.7071067811865476-0.7071067811865476i, 0.7071067811865476+0.7071067811865476i, -0.7071067811865476+0.7071067811865476i, 0.7071067811865476+0.7071067811865476i, -0.7071067811865476+0.7071067811865476i, 0.7071067811865476+0.7071067811865476i, 0.7071067811865476+0.7071067811865476i, 0.7071067811865476+0.7071067811865476i, 0.7071067811865476+0.7071067811865476i, 0.7071067811865476-0.7071067811865476i, 0.7071067811865476+0.7071067811865476i, -0.7071067811865476+0.7071067811865476i, 0.7071067811865476+0.7071067811865476i, -0.7071067811865476+0.7071067811865476i, 0.7071067811865476-0.7071067811865476i, 0.7071067811865476+0.7071067811865476i, -0.7071067811865476+0.7071067811865476i, 0.7071067811865476+0.7071067811865476i, -0.7071067811865476-0.7071067811865476i, 0.7071067811865476-0.7071067811865476i, -0.7071067811865476+0.7071067811865476i, -0.7071067811865476+0.7071067811865476i, -0.7071067811865476+0.7071067811865476i, -0.7071067811865476+0.7071067811865476i, 0.7071067811865476-0.7071067811865476i, 0.7071067811865476+0.7071067811865476i, -0.7071067811865476+0.7071067811865476i, 0.7071067811865476-0.7071067811865476i, -0.7071067811865476-0.7071067811865476i, -0.7071067811865476-0.7071067811865476i, -0.7071067811865476+0.7071067811865476i, 0.7071067811865476+0.7071067811865476i, -0.7071067811865476-0.7071067811865476i, -0.7071067811865476+0.7071067811865476i, -0.7071067811865476-0.7071067811865476i, 0.7071067811865476+0.7071067811865476i, 0.7071067811865476-0.7071067811865476i, 0.7071067811865476+0.7071067811865476i, 0.7071067811865476-0.7071067811865476i, 0.7071067811865476-0.7071067811865476i, 0.7071067811865476+0.7071067811865476i, -0.7071067811865476+0.7071067811865476i, -0.7071067811865476+0.7071067811865476i, -0.7071067811865476+0.7071067811865476i, 0.7071067811865476-0.7071067811865476i, 0.7071067811865476-0.7071067811865476i, -0.7071067811865476+0.7071067811865476i, -0.7071067811865476-0.7071067811865476i, -0.7071067811865476-0.7071067811865476i, 0.7071067811865476-0.7071067811865476i, -0.7071067811865476-0.7071067811865476i, 0.7071067811865476+0.7071067811865476i, 0.7071067811865476-0.7071067811865476i, -0.7071067811865476+0.7071067811865476i, 0.7071067811865476+0.7071067811865476i, 0.7071067811865476-0.7071067811865476i, -0.7071067811865476-0.7071067811865476i, -0.7071067811865476+0.7071067811865476i, -0.7071067811865476-0.7071067811865476i, -0.7071067811865476-0.7071067811865476i, 0.7071067811865476-0.7071067811865476i, -0.7071067811865476+0.7071067811865476i, 0.7071067811865476+0.7071067811865476i, -0.7071067811865476-0.7071067811865476i, -0.7071067811865476+0.7071067811865476i, -0.7071067811865476+0.7071067811865476i, 0.7071067811865476+0.7071067811865476i, -0.7071067811865476-0.7071067811865476i, 0.7071067811865476+0.7071067811865476i, -0.7071067811865476-0.7071067811865476i, 0.7071067811865476+0.7071067811865476i, 0.7071067811865476+0.7071067811865476i, 0.7071067811865476+0.7071067811865476i, -0.7071067811865476+0.7071067811865476i, 0.7071067811865476-0.7071067811865476i, 0.7071067811865476+0.7071067811865476i, -0.7071067811865476-0.7071067811865476i, 0.7071067811865476+0.7071067811865476i, 0.7071067811865476-0.7071067811865476i, 0.7071067811865476-0.7071067811865476i, 0.7071067811865476+0.7071067811865476i, -0.7071067811865476-0.7071067811865476i, -0.7071067811865476+0.7071067811865476i, 0.7071067811865476+0.7071067811865476i, 0.7071067811865476-0.7071067811865476i, -0.7071067811865476-0.7071067811865476i, -0.7071067811865476-0.7071067811865476i, -0.7071067811865476-0.7071067811865476i, 0.7071067811865476-0.7071067811865476i, 0.7071067811865476-0.7071067811865476i, 0.7071067811865476+0.7071067811865476i, 0.7071067811865476-0.7071067811865476i, -0.7071067811865476-0.7071067811865476i, 0.7071067811865476+0.7071067811865476i, -0.7071067811865476+0.7071067811865476i, -0.7071067811865476-0.7071067811865476i, -0.7071067811865476+0.7071067811865476i, -0.7071067811865476+0.7071067811865476i, 0.7071067811865476-0.7071067811865476i, -0.7071067811865476+0.7071067811865476i, -0.7071067811865476+0.7071067811865476i, 0.7071067811865476-0.7071067811865476i, -0.7071067811865476+0.7071067811865476i, -0.7071067811865476-0.7071067811865476i, 0.7071067811865476-0.7071067811865476i, 0.7071067811865476+0.7071067811865476i, -0.7071067811865476-0.7071067811865476i, -0.7071067811865476-0.7071067811865476i, 0.7071067811865476-0.7071067811865476i, -0.7071067811865476-0.7071067811865476i, 0.7071067811865476-0.7071067811865476i, 0.7071067811865476-0.7071067811865476i, 0.7071067811865476+0.7071067811865476i, 0.7071067811865476+0.7071067811865476i, -0.7071067811865476-0.7071067811865476i, -0.7071067811865476+0.7071067811865476i, -0.7071067811865476+0.7071067811865476i, 0.7071067811865476-0.7071067811865476i, -0.7071067811865476-0.7071067811865476i, -0.7071067811865476+0.7071067811865476i, -0.7071067811865476-0.7071067811865476i, -0.7071067811865476+0.7071067811865476i, 0.7071067811865476-0.7071067811865476i, 0.7071067811865476+0.7071067811865476i, 0.7071067811865476+0.7071067811865476i, 0.7071067811865476-0.7071067811865476i, -0.7071067811865476-0.7071067811865476i, -0.7071067811865476+0.7071067811865476i, -0.7071067811865476+0.7071067811865476i, -0.7071067811865476-0.7071067811865476i, -0.7071067811865476-0.7071067811865476i, -0.7071067811865476+0.7071067811865476i, -0.7071067811865476+0.7071067811865476i, -0.7071067811865476+0.7071067811865476i, -0.7071067811865476+0.7071067811865476i, 0.7071067811865476+0.7071067811865476i, 0.7071067811865476+0.7071067811865476i, 0.7071067811865476+0.7071067811865476i, 0.7071067811865476-0.7071067811865476i, 0.7071067811865476-0.7071067811865476i, -0.7071067811865476+0.7071067811865476i, -0.7071067811865476+0.7071067811865476i, -0.7071067811865476+0.7071067811865476i, -0.7071067811865476-0.7071067811865476i, 0.7071067811865476-0.7071067811865476i, -0.7071067811865476+0.7071067811865476i, -0.7071067811865476+0.7071067811865476i, -0.7071067811865476-0.7071067811865476i, -0.7071067811865476+0.7071067811865476i, -0.7071067811865476-0.7071067811865476i, 0.7071067811865476+0.7071067811865476i, 0.7071067811865476+0.7071067811865476i, 0.7071067811865476+0.7071067811865476i, -0.7071067811865476-0.7071067811865476i, 0.7071067811865476-0.7071067811865476i, -0.7071067811865476+0.7071067811865476i, -0.7071067811865476-0.7071067811865476i, -0.7071067811865476+0.7071067811865476i, 0.7071067811865476+0.7071067811865476i, 0.7071067811865476-0.7071067811865476i, -0.7071067811865476+0.7071067811865476i, -0.7071067811865476-0.7071067811865476i, 0.7071067811865476-0.7071067811865476i, 0.7071067811865476-0.7071067811865476i, -0.7071067811865476-0.7071067811865476i, 0.7071067811865476-0.7071067811865476i, 0.7071067811865476-0.7071067811865476i, 0.7071067811865476-0.7071067811865476i, 0.7071067811865476+0.7071067811865476i, 0.7071067811865476-0.7071067811865476i, -0.7071067811865476+0.7071067811865476i, 0.7071067811865476+0.7071067811865476i, 0.7071067811865476+0.7071067811865476i, -0.7071067811865476-0.7071067811865476i, 0.7071067811865476+0.7071067811865476i, -0.7071067811865476-0.7071067811865476i, 0.7071067811865476-0.7071067811865476i, 0.7071067811865476+0.7071067811865476i, -0.7071067811865476+0.7071067811865476i, -0.7071067811865476+0.7071067811865476i, -0.7071067811865476-0.7071067811865476i, 0.7071067811865476-0.7071067811865476i, -0.7071067811865476-0.7071067811865476i, -0.7071067811865476+0.7071067811865476i, 0.7071067811865476-0.7071067811865476i, -0.7071067811865476+0.7071067811865476i, 0.7071067811865476-0.7071067811865476i, 0.7071067811865476-0.7071067811865476i, 0.7071067811865476+0.7071067811865476i, -0.7071067811865476+0.7071067811865476i, -0.7071067811865476-0.7071067811865476i, -0.7071067811865476+0.7071067811865476i, -0.7071067811865476-0.7071067811865476i, 0.7071067811865476-0.7071067811865476i, 0.7071067811865476+0.7071067811865476i, -0.7071067811865476+0.7071067811865476i, -0.7071067811865476-0.7071067811865476i, -0.7071067811865476-0.7071067811865476i, -0.7071067811865476-0.7071067811865476i, -0.7071067811865476-0.7071067811865476i, 0.7071067811865476+0.7071067811865476i, 0.7071067811865476+0.7071067811865476i, -0.7071067811865476+0.7071067811865476i, -0.7071067811865476-0.7071067811865476i, 0.7071067811865476-0.7071067811865476i, -0.7071067811865476-0.7071067811865476i, -0.7071067811865476-0.7071067811865476i, 0.7071067811865476-0.7071067811865476i, 0.7071067811865476+0.7071067811865476i, 0.7071067811865476-0.7071067811865476i, -0.7071067811865476-0.7071067811865476i, 0.7071067811865476-0.7071067811865476i, -0.7071067811865476+0.7071067811865476i, 0.7071067811865476-0.7071067811865476i, -0.7071067811865476+0.7071067811865476i, 0.7071067811865476+0.7071067811865476i, 0.7071067811865476+0.7071067811865476i, -0.7071067811865476+0.7071067811865476i, 0.7071067811865476+0.7071067811865476i, 0.7071067811865476-0.7071067811865476i, 0.7071067811865476-0.7071067811865476i, -0.7071067811865476+0.7071067811865476i, -0.7071067811865476-0.7071067811865476i, -0.7071067811865476+0.7071067811865476i, 0.7071067811865476-0.7071067811865476i, 0.7071067811865476-0.7071067811865476i, 0.7071067811865476+0.7071067811865476i, -0.7071067811865476-0.7071067811865476i, -0.7071067811865476-0.7071067811865476i, 0.7071067811865476+0.7071067811865476i, -0.7071067811865476-0.7071067811865476i, -0.7071067811865476-0.7071067811865476i, 0.7071067811865476-0.7071067811865476i, -0.7071067811865476+0.7071067811865476i, 0.7071067811865476-0.7071067811865476i, -0.7071067811865476-0.7071067811865476i, 0.7071067811865476+0.7071067811865476i, -0.7071067811865476+0.7071067811865476i, -0.7071067811865476+0.7071067811865476i, -0.7071067811865476+0.7071067811865476i, 0.7071067811865476+0.7071067811865476i, 0.7071067811865476-0.7071067811865476i, 0.7071067811865476+0.7071067811865476i, -0.7071067811865476-0.7071067811865476i, 0.7071067811865476-0.7071067811865476i, 0.7071067811865476+0.7071067811865476i, -0.7071067811865476-0.7071067811865476i, -0.7071067811865476+0.7071067811865476i, 0.7071067811865476-0.7071067811865476i, 0.7071067811865476-0.7071067811865476i, 0.7071067811865476-0.7071067811865476i, -0.7071067811865476-0.7071067811865476i, 0.7071067811865476-0.7071067811865476i, 0.7071067811865476+0.7071067811865476i, 0.7071067811865476-0.7071067811865476i, -0.7071067811865476+0.7071067811865476i, 0.7071067811865476-0.7071067811865476i, 0.7071067811865476+0.7071067811865476i, 0.7071067811865476-0.7071067811865476i, 0.7071067811865476+0.7071067811865476i, 0.7071067811865476-0.7071067811865476i, 0.7071067811865476+0.7071067811865476i, 0.7071067811865476+0.7071067811865476i, 0.7071067811865476+0.7071067811865476i, -0.7071067811865476+0.7071067811865476i, 0.7071067811865476+0.7071067811865476i, 0.7071067811865476+0.7071067811865476i, 0.7071067811865476-0.7071067811865476i, 0.7071067811865476+0.7071067811865476i, -0.7071067811865476-0.7071067811865476i, 0.7071067811865476+0.7071067811865476i, 0.7071067811865476+0.7071067811865476i, 0.7071067811865476-0.7071067811865476i, -0.7071067811865476+0.7071067811865476i, -0.7071067811865476-0.7071067811865476i, 0.7071067811865476+0.7071067811865476i, 0.7071067811865476-0.7071067811865476i, 0.7071067811865476-0.7071067811865476i, 0.7071067811865476-0.7071067811865476i, -0.7071067811865476-0.7071067811865476i, 0.7071067811865476+0.7071067811865476i, 0.7071067811865476+0.7071067811865476i, -0.7071067811865476-0.7071067811865476i, -0.7071067811865476+0.7071067811865476i, -0.7071067811865476-0.7071067811865476i, 0.7071067811865476-0.7071067811865476i, 0.7071067811865476-0.7071067811865476i, -0.7071067811865476+0.7071067811865476i, 0.7071067811865476-0.7071067811865476i, -0.7071067811865476-0.7071067811865476i, 0.7071067811865476-0.7071067811865476i, -0.7071067811865476+0.7071067811865476i, 0.7071067811865476+0.7071067811865476i, -0.7071067811865476+0.7071067811865476i, -0.7071067811865476+0.7071067811865476i, 0.7071067811865476+0.7071067811865476i, 0.7071067811865476+0.7071067811865476i, 0.7071067811865476-0.7071067811865476i, 0.7071067811865476-0.7071067811865476i, -0.7071067811865476-0.7071067811865476i, -0.7071067811865476+0.7071067811865476i, 0.7071067811865476+0.7071067811865476i, -0.7071067811865476-0.7071067811865476i, -0.7071067811865476-0.7071067811865476i, -0.7071067811865476-0.7071067811865476i, -0.7071067811865476+0.7071067811865476i, 0.7071067811865476-0.7071067811865476i, -0.7071067811865476+0.7071067811865476i, 0.7071067811865476+0.7071067811865476i, 0.7071067811865476-0.7071067811865476i, -0.7071067811865476+0.7071067811865476i, -0.7071067811865476+0.7071067811865476i, 0.7071067811865476-0.7071067811865476i]
  out "symbols":cdb[](array[numeric]) format="%.3f"
  out "output bit stream":i8[](array[numeric])
  out "output array":cdb[][](array[numeric])
  out "Total Size":i32
  in  "text":string
  out "appended array":i8[](array[numeric])
  out "Output Complex Data":cdb[](array[numeric])
  in  "Tab Control":enum32{"Parameters", "Debug"}(tab)
  in  "device names":refnum<k15>="192.168.10.2"
  in  "IQ rate 2":dbl=5000000.0 format="%#_6p"
  in  "gain 2":dbl=9.0 format="%#_6f"
  in  "carrier frequency":dbl=910000000.0 format="%#_6p"
  out "coerced IQ rate":dbl=100000.0 format="%#_6p"
  in  "active antenna":string="TX1"
  in  "error in (no error)":errorcluster
  out "error out":errorcluster
  out "millisecond timer value 2":u32
  out "Power Spectrum / PSD":cluster{"f0":dbl, "df":dbl, "magnitude":dbl[]} {"magnitude" format="%.2p"; "f0" format="%0.2p"; "df" format="%0.2p"}
  out "SNR":dbl
  out "x/y":dbl
  in  "IQ rate":dbl=100000.0 format="%#_6p"
  in  "gain":dbl format="%#_6f"
  out "CH1 is Free":bool
  # "Guard\nBand"
  # "Sync\nSeq"
  # "Packet\nNumber"
  # "Pad\nData"
  # "Blank\nFrame"
  # "Data"
types:
  T1 = cluster{"Samples per Symbol":i32, "symbol map":cdb[], "Differential PSK":enum16{"disable", "enable"}, "PSK type":u16}
  T2 = enum32{"Specify Message", "Specify Packet", "Specify Modulation", "Tx Parameters", "Debug"}
  T3 = cluster{"Guard Bits ":i32, "Sync Bits":i32, "Message Bits":i32}
  T4 = cluster{"Alpha":dbl, "Filter Length":i32, "TX Filter":enum16{"none", "Raised Cosine", "Root Raised Cos", "Gaussian"}}
  T5 = cluster{"Tx IQ Sampling\nRate [s/sec]":dbl, "Tx Frequency [Hz]":dbl, "Tx Gain [dB]":dbl, "Tx Antenna":string}
  T6 = cluster{"Decimated Array":dbl[], "Decimated Array":dbl[]}[]
  T7 = cluster{"samples per symbol (16)":i32, "symbol map":cdb[], "differential PSK":enum16{"disable", "enable"}, "PSK type":u16}
  T8 = cluster{"s? t:f":cluster{"t0":dbl, "dt":dbl, "Y":cdb[]}, i32}
  T9 = cluster{"output complex waveform":cluster{"t0":dbl, "dt":dbl, "Y":cdb[]}, i32}
  T10 = cluster{"constellation":dbl[], "oversampled data":dbl[]}[]
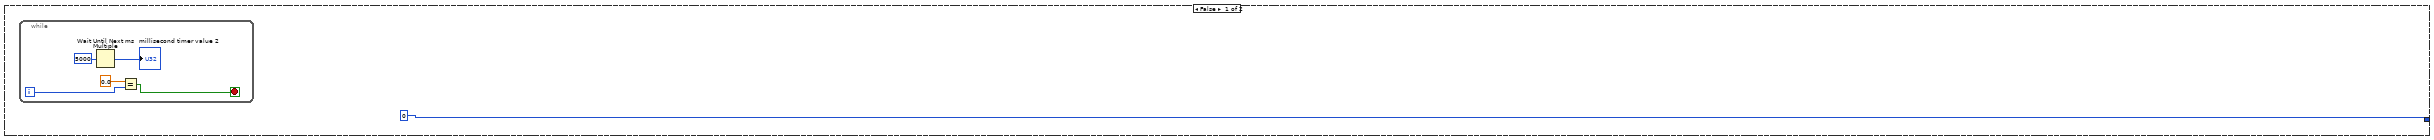
[diagram p3: hidden frame]
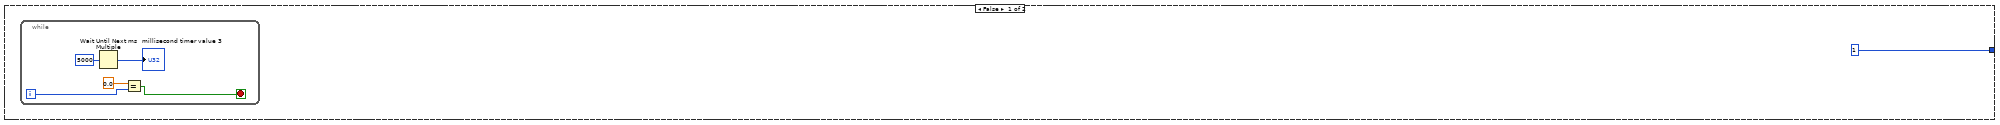
[diagram p4: hidden frame]
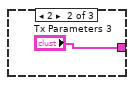
[diagram p5: hidden frame]
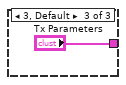
[diagram p6: hidden frame]
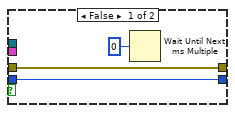
[diagram p7: hidden frame]
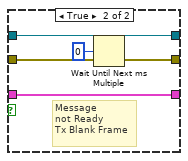
[diagram p8: hidden frame]
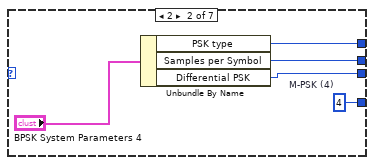
[diagram p9: hidden frame]
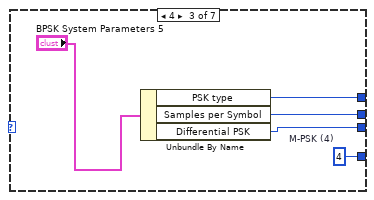
[diagram p10: hidden frame]
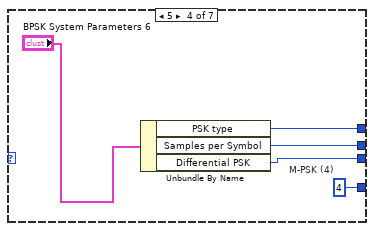
[diagram p11: hidden frame]
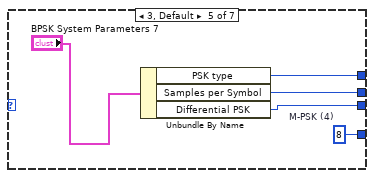
[diagram p12: hidden frame]
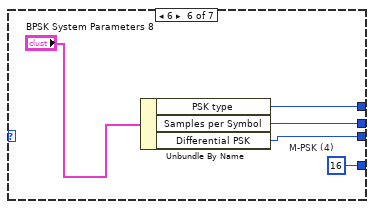
[diagram p13: hidden frame]
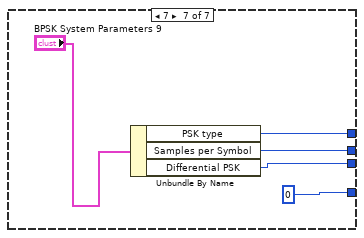
[diagram p14: hidden frame]
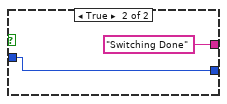
[diagram p15: hidden frame]
diagram:
  n1 = flat-sequence {
    tunnel: w3 -> [w9]
    tunnel: [w7] -> w2
    tunnel: w1 -> [w6]
    tunnel: [w132] -> w5
    tunnel: w5 -> [w202]
    tunnel: [w201] -> w4
    frame #0 {
      n2 = Or(x=w9, y=w6) -> (x .or. y?=w8:i32)
      n3 = case shown="0, Default" w8 {
        tunnel: [w11 _] -> w10
        frame 0, Default {
          n4 = call <instrlib>:"niUSRP Open Rx Session.vi"("device names"=refnum<k15> "192.168.10.2") -> ("session handle out"=w16:refnum<k15>, "error out"=w15:errorcluster)  [unwired: 13 in]
          n5 = while {
            tunnel: w16 -> [w46]
            tunnel: w15 -> [w43]
            tunnel: [w29] -> w13
            tunnel: [w28] -> w12
            tunnel: [w17] -> w11
            i -> [w20]
            stop <- w19 stop-if-true
            w25 = 3.82195e-05 ("y")
            n6 = Equal?(x=1, y=w20) -> (x = y?=w19:bool)
            n7 = call <instrlib>:"niUSRP Configure Signal.vi"("session handle"=w46, "IQ rate"="IQ rate", "carrier frequency"=470000000.0, "gain"="gain", "error in (no error)"=w43, "active antenna"="RX1") -> ("session handle out"=w45:refnum<k15>, "error out"=w44:errorcluster)  [unwired: 5 in, 3 out]
            n8 = call <instrlib>:"niUSRP Initiate.vi"("session handle"=w45, "error in (no error)"=w44) -> ("session handle out"=w42:refnum<k15>, "error out"=w41:errorcluster)  [unwired: 12 in]
            n9 = while {
              tunnel: w42 -> [w65]
              shift-right: [w49] -> w40
              shift-left: w41 -> [w62]
              tunnel: [w64] -> w39
              shift-right: [w47] -> _
              shift-left: _ -> [w63]
              shift-right: [w56] -> w37
              shift-left: 0.0 -> [w57]
              tunnel: [w51] -> w36
              tunnel: 1000 -> [w54]
              i -> [w51]
              stop <- w50 stop-if-true
              n10 = call-poly <instrlib>:"niUSRP Fetch Rx Data (poly).vi"("session handle"=w65, "number of samples"=w54, "error in (no error)"=w62) -> ("session handle out"=w64:refnum<k15>, "data"=w48:cluster{"t0":dbl, "dt":dbl, "Y":cdb[]}, "error out"=w49:errorcluster)  [unwired: 9 in, 1 out]
              n11 = call-poly <vilib>:"FFT Power Spectrum and PSD.vi"("error in (no error)"=w62, "time signal"=w63) -> ("Power Spectrum / PSD"=w61:cluster{"f0":dbl, "df":dbl, "magnitude":dbl[]})  [unwired: 6 in, 3 out]
              "Power Spectrum / PSD" <- w61
              n12 = Unbundle By Name(w61) -> ("magnitude"=w60:dbl[])
              n13 = Unbundle By Name(w48) -> ("Y"=w47:cdb[])
              n14 = Build Array(w60) -> (w59:dbl[][])
              n15 = Array Subset(array=w59, length (col)=1000 ("length")) -> (w58:dbl[][])  [unwired: 3 in]
              n16 = Equal?(x=1000, y=w51) -> (x = y?=w50:bool)
              n17 = Add Array Elements(numeric array=w58) -> (sum=w55:dbl)
              n18 = Add(x=w55, y=w57) -> (x+y=w56:dbl)
            }
            n19 = Divide(x=w37, y=w36) -> (x/y=w22:dbl)
            n20 = call <instrlib>:"niUSRP Abort.vi"("session handle"=w39, "error in (no error)"=w40) -> ("session handle out"=w29:refnum<k15>, "error out"=w28:errorcluster)  [unwired: 12 in]
            n21 = Subtract(x=w22, y=w25) -> (x-y=w24:dbl)
            n22 = Less?(x=w22, y=3.82195e-05) -> (x < y?=w17:bool)
            "CH1 is Free" <- w17
            n23 = Divide(x=w24, y=w25) -> (x/y=w35:dbl)
            "x/y" <- w35
            n24 = Logarithm Base 10(1:w35) -> (0:w34:dbl)
            n25 = Multiply(x=w34, y=10.0) -> (x*y=→"SNR":dbl)
          }
          n26 = call <instrlib>:"niUSRP Close Session.vi"("session handle"=w13, "error in (no error)"=w12) -> ()  [unwired: 13 in, 1 out]
        }
        frame 1 {
        }
      }
      n27 = case shown="True" w10 {
        tunnel: [0 _] -> w7
        frame False {
          n28 = while {
            i -> [w69]
            stop <- w68 stop-if-true
            n29 = Wait Until Next ms Multiple(millisecond multiple=u32 5000) -> (millisecond timer value=→"millisecond timer value 2":u32)
            n30 = Equal?(x=0.0, y=w69) -> (x = y?=w68:bool)
          }
        }
        frame True {
          w81 = cdb[] [0.7071067811865476+0.7071067811865476i, 0.7071067811865476-0.7071067811865476i, -0.7071067811865476+0.7071067811865476i, -0.7071067811865476-0.7071067811865476i]  # 4QAM MAP
          # "1."
          n31 = call <instrlib>:"niUSRP Open Tx Session.vi"("device names"="device names", "reset"=TRUE, "error in (no error)"="error in (no error)") -> ("session handle out"=w78:refnum<k15>, "error out"=w79:errorcluster)  [unwired: 11 in]
          n32 = Add(x="IQ rate 2", y="carrier frequency") -> (x+y=w73:dbl)
          n33 = property class="niUSRP"(reference=w78, error in=w79, "LO Frequency"=w73) -> (reference out=w82:refnum<k15>, error out=w80:errorcluster)
          n34 = call <instrlib>:"niUSRP Configure Signal.vi"("session handle"=w82, "IQ rate"="IQ rate 2", "carrier frequency"="carrier frequency", "gain"="gain 2", "error in (no error)"=w80, "active antenna"="active antenna") -> ("session handle out"=w77:refnum<k15>, "coerced IQ rate"=→"coerced IQ rate":dbl)  [unwired: 5 in, 3 out]
          n35 = while {
            tunnel: w77 -> [w109]
            tunnel: [w108] -> w89
            tunnel: [w107] -> w88
            tunnel: w81 -> [w106]
            stop <- "stop 2" stop-if-true
            w105 = 125 ("y")
            # "10."
            # "8"
            # "3"
            # "2."
            # "1"
            n36 = String To Byte Array(string="text") -> (unsigned byte array=w98:u8[])
            n37 = for {
              tunnel: w98 -> [w114] mode=indexing
              tunnel: [w112] -> w97 mode=indexing
              n38 = Number To Boolean Array(number=w114) -> (Boolean array=w113:bool[])
              n39 = Boolean To (0,1)(Boolean=w113) -> (0, 1=w112:i16[])
            }
            n40 = To Byte Integer(number=w97) -> (8bit integer=w94:i8[][])
            n41 = Array Size(array=w94) -> (size(s)=w96:i32[])
            n42 = Multiply Array Elements(1:w96) -> (0:w95:i32)
            n43 = Reshape Array(w94, w95) -> (w93:i8[])
            "output bit stream" <- w93
            "appended array" <- w93
            n44 = call-poly <vilib>:"MT Map Bits to Symbols.vi"("input bit stream"=w93, "symbol map"=w106) -> ("symbols"=w92:cdb[], "error out"=w104:errorcluster)  [unwired: 12 in]
            "Outgoing Constellation" <- w92
            "symbols" <- w92
            n45 = Array Size(array=w92) -> (size(s)=w111:i32)
            n46 = Divide(x=w111, y=w105) -> (x/y=w110:dbl)
            n47 = Reshape Array(w92, w110, w105) -> (w91:cdb[][])
            "output array" <- w91
            n48 = for {
              tunnel: w91 -> [w122] mode=indexing
              tunnel: [w116] -> w102 mode=concatenating
              w123 = cdb[] [-0.7071067811865475-0.7071067811865475i, -0.7071067811865475-0.7071067811865475i, -0.7071067811865475-0.7071067811865475i, 0.7071067811865475-0.7071067811865475i, 0.7071067811865475-0.7071067811865475i, 0.7071067811865475+0.7071067811865475i, 0.7071067811865475-0.7071067811865475i, -0.7071067811865475-0.7071067811865475i, 0.7071067811865475+0.7071067811865475i, -0.7071067811865475+0.7071067811865475i, -0.7071067811865475-0.7071067811865475i, -0.7071067811865475+0.7071067811865475i, -0.7071067811865475+0.7071067811865475i, 0.7071067811865475-0.7071067811865475i, -0.7071067811865475+0.7071067811865475i, -0.7071067811865475+0.7071067811865475i, 0.7071067811865475-0.7071067811865475i, -0.7071067811865475+0.7071067811865475i, -0.7071067811865475-0.7071067811865475i, 0.7071067811865475-0.7071067811865475i, 0.7071067811865475+0.7071067811865475i, -0.7071067811865475-0.7071067811865475i, -0.7071067811865475-0.7071067811865475i, 0.7071067811865475-0.7071067811865475i, -0.7071067811865475-0.7071067811865475i, 0.7071067811865475-0.7071067811865475i, 0.7071067811865475-0.7071067811865475i, 0.7071067811865475+0.7071067811865475i, 0.7071067811865475+0.7071067811865475i, -0.7071067811865475-0.7071067811865475i, -0.7071067811865475+0.7071067811865475i, -0.7071067811865475+0.7071067811865475i, 0.7071067811865475-0.7071067811865475i, -0.7071067811865475-0.7071067811865475i, -0.7071067811865475+0.7071067811865475i, -0.7071067811865475-0.7071067811865475i, -0.7071067811865475+0.7071067811865475i, 0.7071067811865475-0.7071067811865475i, 0.7071067811865475+0.7071067811865475i, 0.7071067811865475+0.7071067811865475i, 0.7071067811865475-0.7071067811865475i, -0.7071067811865475-0.7071067811865475i, -0.7071067811865475+0.7071067811865475i, -0.7071067811865475+0.7071067811865475i, -0.7071067811865475-0.7071067811865475i, -0.7071067811865475-0.7071067811865475i, -0.7071067811865475+0.7071067811865475i, -0.7071067811865475+0.7071067811865475i, -0.7071067811865475+0.7071067811865475i, -0.7071067811865475+0.7071067811865475i]  # Reference Symbols
              # "7"
              # "6"
              # "5"
              # "4"
              n49 = Array Size(array=w122) -> (size(s)=→"Data Size":i32)
              n50 = call "Data Reference Interleave.vi"("Data Symbols"=w122, "Reference Symbols"=w123) -> ("Interleaved Output"=w120:cdb[])  [unwired: 9 in]
              "Interleaved Output" <- w120
              n51 = Array Size(array=w120) -> (size(s)=→"Reference Symbols \n         Added":i32)
              n52 = call "Zero Padding.vi"("Array in"=w120) -> ("Array out"=w118:cdb[])  [unwired: 10 in]
              "Array out" <- w118
              n53 = Array Size(array=w118) -> (size(s)=→"After Zero \n  Padding":i32)
              n54 = call-poly <vilib>:"Inverse FFT.vi"("shift?"=TRUE, "FFT {X}"=w118) -> ("X"=w124:cdb[])  [unwired: 8 in, 1 out]
              "X" <- w124
              n55 = call "CP Insertion.vi"("Input"=w124) -> ("Output with CP"=w116:cdb[])  [unwired: 10 in]
              "Output with CP" <- w116
              n56 = Array Size(array=w116) -> (size(s)=→"After CP":i32)
            }
            n57 = Multiply(x=w102, y=0.5 ("value")) -> (x*y=w101:cdb[])
            "Output Complex Data" <- w101
            n58 = Array Size(array=w101) -> (size(s)=→"Total Size":i32)
            n59 = call-poly <instrlib>:"niUSRP Write Tx Data (poly).vi"("session handle"=w109, "data"=w101, "error in (no error)"=w104) -> ("session handle out"=w107:refnum<k15>, "error out"=w108:errorcluster)  [unwired: 11 in]
          }
          n60 = call <instrlib>:"niUSRP Close Session.vi"("session handle"=w88, "error in (no error)"=w89) -> ("error out"=→"error out":errorcluster)  [unwired: 13 in]
        }
      }
    }
    frame #1 {
      n61 = while {
        i -> [w128]
        stop <- w127 stop-if-true
        n62 = Wait Until Next ms Multiple(millisecond multiple=u32 5000) -> (millisecond timer value=→"millisecond timer value":u32)
        n63 = Equal?(x=0.0, y=w128) -> (x = y?=w127:bool)
      }
    }
    frame #2 {
      (unwired) TRUE ("number of samples is finite")
      # "1."
      n64 = call <instrlib>:"niUSRP Open Rx Session.vi"("device names"=refnum<k15> "192.168.10.2", "error in (no error)"=errorcluster {"status"=FALSE, "code"=0, "source"=""}) -> ("session handle out"=w143:refnum<k15>, "error out"=w142:errorcluster)  [unwired: 12 in]
      n65 = call <instrlib>:"niUSRP Configure Signal.vi"("session handle"=w143, "IQ rate"="IQ rate 3", "carrier frequency"="Carrier frequency", "gain"="Gain", "error in (no error)"=w142, "active antenna"="Active antenna") -> ("session handle out"=w145:refnum<k15>, "coerced IQ rate"=w146:dbl, "error out"=w144:errorcluster)  [unwired: 5 in, 2 out]
      "Coerced IQ rate" <- w146
      n66 = call <instrlib>:"niUSRP Initiate.vi"("session handle"=w145, "error in (no error)"=w144) -> ("session handle out"=w158:refnum<k15>, "error out"=w157:errorcluster)  [unwired: 12 in]
      n67 = while {
        tunnel: w158 -> [w175]
        tunnel: w157 -> [w170]
        tunnel: [w174] -> w149
        tunnel: "Number of samples" -> [w171]
        tunnel: w146 -> [w177]
        tunnel: [w176] -> w152
        tunnel: [w159] -> w140
        i -> [w161]
        stop <- w162 stop-if-true
        # "2."
        # "3."
        n68 = call-poly <instrlib>:"niUSRP Fetch Rx Data (poly).vi"("session handle"=w175, "number of samples"=w171, "error in (no error)"=w170) -> ("session handle out"=w174:refnum<k15>, "data"=w172:cdb[], "error out"=w173:errorcluster)  [unwired: 9 in, 1 out]
        "error out 2" <- w173
        n69 = call "VanDeBeek.vi"("Input"=w172) -> ("Phase"=→"Phase":dbl[], "Magnitude"=→"Magnitude":dbl[], "Indices"=w167:i32[], "CFOest (Hz)"=w166:dbl[])  [unwired: 6 in, 1 out]
        n70 = Divide(x=w177, y=256.0 ("x")) -> (x/y=w168:dbl)
        n71 = Multiply(x=w166, y=w168) -> (x*y=w163:dbl[])
        "CFOest (Hz)" <- w163
        n72 = for {
          tunnel: w163 -> [w192]
          workers-P: _ -> [_]
          tunnel: w177 -> [w191]
          tunnel: w173 -> [w190]
          tunnel: [w189] -> w176
          tunnel: w167 -> [w184] mode=indexing
          tunnel: w172 -> [w187]
          tunnel: [w181] -> w159 mode=indexing
          i -> [w182]
          w183 = 256  # N-Point FFT Size
          w186 = 64  # CP Size
          w194 = cdb[] [0.7071067811865476+0.7071067811865476i, 0.7071067811865476-0.7071067811865476i, -0.7071067811865476+0.7071067811865476i, -0.7071067811865476-0.7071067811865476i]  # 4QAM MAP
          w185 = 320  # Frame
          # "10."
          # "9."
          # "8."
          # "7."
          # "6."
          # "5."
          # "4."
          n73 = call "CP Removal.vi"("Input"=w187, "Indicies"=w184, "i"=w182, "Frame Size"=w185, "CP Size"=w186, "N-Point FFT Size"=w183) -> ("Output Without CP"=w188:cdb[])  [unwired: 9 in]
          n74 = call "CFO Correction.vi"("fs"=w191, "CFOest (freq)"=w192, "Index"=w182, "Input"=w188) -> ("Output"=w195:cdb[])  [unwired: 7 in]
          n75 = call-poly <vilib>:"FFT.vi"("FFT size"=256, "shift?"=TRUE, "X"=w195) -> ("FFT {X}"=w196:cdb[])  [unwired: 7 in, 1 out]
          n76 = Complex To Polar(r * e^(i*theta)=w196) -> (r=→"FFT {X}":dbl[], theta=→"theta":dbl[])
          n77 = call "Zero Pad Removal and Deinterleave.vi"("Input"=w196) -> ("Ref"=w180:cdb[], "Data"=w178:cdb[])  [unwired: 9 in]
          "Unequalized Data" <- w178
          n78 = call "Channel Estimation Linear.vi"("Ref"=w180) -> ("Hest"=w179:cdb[])  [unwired: 10 in]
          n79 = Multiply(x=w178, y=w179) -> (x*y=w193:cdb[])
          "Equalized Data" <- w193
          n80 = call-poly <vilib>:"MT Map Symbols to Bits.vi"("symbols"=w193, "symbol map"=w194, "error in (no error)"=w190) -> ("output bit stream"=w181:i8[], "error out"=w189:errorcluster)  [unwired: 11 in]
          "Output bit stream" <- w181
        }
        "output bit stream 2" <- w159
        n81 = Equal?(x=4, y=w161) -> (x = y?=w162:bool)
      }
      "output bit stream 3" <- w140
      n82 = call <instrlib>:"niUSRP Abort.vi"("session handle"=w149, "error in (no error)"=w152) -> ("session handle out"=w150:refnum<k15>, "error out"=w151:errorcluster)  [unwired: 12 in]
      n83 = Reshape Array(w140, 16 ("dimension size")) -> (w138:i8[])
      n84 = call <instrlib>:"niUSRP Close Session.vi"("session handle"=w150, "error in (no error)"=w151) -> ("error out"=→"error out 3":errorcluster)  [unwired: 13 in]
      n85 = Subtract(x=w138, y="Reference Array") -> (x-y=w136:dbl[])
      n86 = Absolute Value(x=w136) -> (abs(x)=w135:dbl[])
      n87 = Add Array Elements(numeric array=w135) -> (sum=w133:dbl)
      n88 = Equal?(x=0.0, y=w133) -> (x = y?=w132:bool)
    }
    frame #3 {
      n89 = case shown="True" w202 {
        tunnel: [1 _] -> w201
        frame False {
          n90 = while {
            i -> [w206]
            stop <- w205 stop-if-true
            n91 = Wait Until Next ms Multiple(millisecond multiple=u32 5000) -> (millisecond timer value=→"millisecond timer value 3":u32)
            n92 = Equal?(x=0.0, y=w206) -> (x = y?=w205:bool)
          }
        }
        frame True {
          n93 = flat-sequence {
            tunnel: ["Enter control signal (1,2 or 3)\n1. Power\n2. Trade Off\n3. Bandwidth"] -> w213
            tunnel: w209 -> [w216]
            tunnel: w213 -> [w378]
            tunnel: [w380] -> w212
            tunnel: [w379] -> w211
            tunnel: w212 -> [w399]
            tunnel: w211 -> [w398]
            tunnel: [w397] -> w210
            frame #0 {
              n94 = case shown="1" w216 {
                tunnel: ["Tx Parameters 2" "Tx Parameters 3" "Tx Parameters"] -> w215
                frame 1 {
                }
                frame 2 {
                }
                frame 3, Default {
                }
              }
              n95 = case shown="1" w216 {
                tunnel: [w344 w349 w356 w361 w366 w372 w375] -> w219
                tunnel: [w345 w350 w355 w360 w365 w371 w376] -> w245
                tunnel: [w347 w352 w357 w362 w364 w370 0 ("M-PSK (4)")] -> w236
                tunnel: [w346 w351 w354 w359 w367 w369 w377] -> w225
                frame 1 {
                  w347 = 2  # M-PSK
                  n96 = Unbundle By Name("BPSK System Parameters 3") -> ("PSK type"=w346:u16, "Samples per Symbol"=w344:i32, "Differential PSK"=w345:enum16{"disable", "enable"})
                }
                frame 2 {
                  w352 = 4  # M-PSK (4)
                  n97 = Unbundle By Name("BPSK System Parameters 4") -> ("PSK type"=w351:u16, "Samples per Symbol"=w349:i32, "Differential PSK"=w350:enum16{"disable", "enable"})
                }
                frame 4 {
                  w357 = 4  # M-PSK (4)
                  n98 = Unbundle By Name("BPSK System Parameters 5") -> ("PSK type"=w354:u16, "Samples per Symbol"=w356:i32, "Differential PSK"=w355:enum16{"disable", "enable"})
                }
                frame 5 {
                  w362 = 4  # M-PSK (4)
                  n99 = Unbundle By Name("BPSK System Parameters 6") -> ("PSK type"=w359:u16, "Samples per Symbol"=w361:i32, "Differential PSK"=w360:enum16{"disable", "enable"})
                }
                frame 3, Default {
                  w364 = 8  # M-PSK (4)
                  n100 = Unbundle By Name("BPSK System Parameters 7") -> ("PSK type"=w367:u16, "Samples per Symbol"=w366:i32, "Differential PSK"=w365:enum16{"disable", "enable"})
                }
                frame 6 {
                  w370 = 16  # M-PSK (4)
                  n101 = Unbundle By Name("BPSK System Parameters 8") -> ("PSK type"=w369:u16, "Samples per Symbol"=w372:i32, "Differential PSK"=w371:enum16{"disable", "enable"})
                }
                frame 7 {
                  n102 = Unbundle By Name("BPSK System Parameters 9") -> ("PSK type"=w377:u16, "Samples per Symbol"=w375:i32, "Differential PSK"=w376:enum16{"disable", "enable"})
                }
              }
              "M-PSK (4)" <- w236
              n103 = call <instrlib>:"niUSRP Open Tx Session.vi"("device names"="USRP IP address", "reset"=TRUE) -> ("session handle out"=w229:refnum<k15>, "error out"=w228:errorcluster)  [unwired: 12 in]
              n104 = call "subCallConfigTx.vi"("session handle"=w229, "Tx Parameters"=w215, "error in"=w228) -> ("session handle out"=w235:refnum<k15>, "Actual Tx Parameters"=w234:T5, "error out"=w238:errorcluster)  [unwired: 10 in]
              "Actual Tx Parameters" <- w234
              n105 = Unbundle By Name(w234) -> ("Tx IQ Sampling\nRate [s/sec]"=w220:dbl)
              n106 = call-poly <vilib>:"MT Generate System Parameters.vi"("samples per symbol (16)"=w219, "PSK type"=w225, "M-PSK (4)"=w236, "differential PSK"=w245) -> ("PSK system parameters"=w226:T7)  [unwired: 9 in, 2 out]
              n107 = call "subGeneratePackets.vi"("Samples per Symbol"=w219, "Packet Pad \n[samples]"="Packet Pad \n[samples]", "PSK system parameters"=w226, "Tx IQ Sampling\nRate [s/sec]"=w220, "Pulse Shaping Filter Parameters"="Pulse Shaping Filter Parameters", "Packet Repeat"="Packet Repeat", "PN sequence order\nfor Sync Bits"="PN sequence order\nfor Sync Bits", "Packet Parameters"="Packet Parameters", "Message Text"="Enter control signal (1,2 or 3)\n1. Power\n2. Trade Off\n3. Bandwidth") -> ("Number of Packets"=w233:i32, "Packets"=w239:cluster{"t0":dbl, "dt":dbl, "Y":cdb[]}[], "Symbol Rate"=→"Symbol Rate\n[symbols/sec]":dbl)  [unwired: 4 in]
              "Number of Packets in Message" <- w233
              n108 = Reciprocal(x=w220) -> (1/x=w237:dbl)
              n109 = Bundle("s? t:f"=cluster{"t0":dbl, "dt":dbl, "Y":cdb[]} {"t0"=0.0, "dt"=0.0, "Y"=[]}, 0) -> (w241:T8)  [unwired: 1 in]
              n110 = while {
                tunnel: cdb 0.0+0.0i ("element") -> [w273]
                tunnel: "Blank Frame \n[samples]" -> [w272]
                tunnel: w241 -> [w266]
                tunnel: "Queue Length" -> [w264]
                tunnel: w239 -> [w263]
                tunnel: w238 -> [w262]
                tunnel: w237 -> [w259]
                tunnel: w235 -> [w258]
                tunnel: w233 -> [w257]
                tunnel: [w252] -> w224
                tunnel: w219 -> [w251]
                stop <- w249 stop-if-true
                n111 = Obtain Queue(max queue size (-1, unlimited)=w264, element data type=w266) -> (queue out=w271:refnum<queue>, error out=w255:errorcluster)  [unwired: 3 in, 1 out]
                n112 = Initialize Array(w273, w272) -> (w270:cdb[])
                n113 = Bundle By Name(cluster=cluster{"t0":dbl, "dt":dbl, "Y":cdb[]} {"t0"=0.0, "dt"=0.0, "Y"=[]} ("s? t:f"), "dt"=w259, "Y"=w270) -> (w269:cluster{"t0":dbl, "dt":dbl, "Y":cdb[]})
                n114 = while {
                  tunnel: w258 -> [w323]
                  shift-right: [w314] -> w261
                  shift-left: w262 -> [w324]
                  tunnel: w271 -> [w332]
                  tunnel: w269 -> [w329]
                  tunnel: [w328] -> w268
                  tunnel: [w322] -> w260
                  shift-right: [w319] -> w267
                  shift-left: w255 -> [w325]
                  i -> [w316]
                  stop <- w312 stop-if-true
                  n115 = Get Queue Status(queue=w332, error in (no error)=w325) -> (queue out=w327:refnum<queue>, error out=w326:errorcluster, # elements in queue=w331:i32)  [unwired: 1 in, 5 out]
                  n116 = Equal To 0?(x=w331) -> (x = 0?=w330:bool)
                  n117 = case shown="False" w330 {
                    tunnel: w329 -> [_ w342]
                    tunnel: [w334 w342] -> w317
                    tunnel: [w338 w340] -> w328
                    tunnel: [w333 w341] -> w319
                    tunnel: w327 -> [w337 w340]
                    tunnel: w326 -> [w336 w341]
                    frame False {
                      n118 = Dequeue Element(queue=w337, error in (no error)=w336) -> (queue out=w338:refnum<queue>, element=w335:T8, error out=w333:errorcluster)  [unwired: 1 in, 1 out]
                      n119 = Unbundle(w335) -> ("s? t:f"=w334:cluster{"t0":dbl, "dt":dbl, "Y":cdb[]})  [unwired: 1 out]
                    }
                    frame True {
                      # "Message\nnot Ready\nTx Blank Frame"
                      n120 = Wait Until Next ms Multiple(millisecond multiple=u32 0) -> ()  [unwired: 1 out]
                    }
                  }
                  n121 = Unbundle By Name(w319) -> ("status"=w318:bool)
                  n122 = call-poly <instrlib>:"niUSRP Write Tx Data (poly).vi"("session handle"=w323, "data"=w317, "end of data?"="stop", "error in (no error)"=w324) -> ("session handle out"=w322:refnum<k15>, "error out"=w314:errorcluster)  [unwired: 10 in]
                  n123 = Unbundle By Name(w314) -> ("status"=w321:bool)
                  n124 = Equal?(x=1, y=w316) -> (x = y?=w313:bool)
                  n125 = Compound Arithmetic op=OR(w318, w321, "stop", w313) -> (w312:bool)
                  "result" <- w312
                }
                n126 = while {
                  tunnel: w271 -> [w302]
                  shift-right: [w295] -> _
                  shift-left: 0 -> [w291]
                  tunnel: w263 -> [w292]
                  tunnel: w264 -> [w294]
                  tunnel: w257 -> [w293]
                  shift-right: [w283] -> _
                  shift-left: w255 -> [w297]
                  tunnel: w251 -> [w287]
                  i -> [w280]
                  stop <- w282 stop-if-true
                  n127 = Quotient & Remainder(x=w291, y=w293) -> (x-y*floor(x/y)=w290:i32)  [unwired: 1 out]
                  n128 = Index Array(array=w292, index=w290) -> (element=w285:cluster{"t0":dbl, "dt":dbl, "Y":cdb[]})
                  n129 = Get Queue Status(queue=w302, error in (no error)=w297) -> (queue out=w301:refnum<queue>, error out=w298:errorcluster, # elements in queue=w300:i32)  [unwired: 1 in, 5 out]
                  n130 = Less?(x=w300, y=w294) -> (x < y?=w299:bool)
                  n131 = Bundle("output complex waveform"=w285, w290) -> (w296:T9)  [unwired: 1 in]
                  n132 = case shown="True" w299 {
                    tunnel: w298 -> [w303 w311]
                    tunnel: w301 -> [_ w310]
                    tunnel: [w303 w309] -> w283
                    tunnel: w296 -> [_ w308]
                    tunnel: w291 -> [w305 w307]
                    tunnel: [w305 w306] -> w295
                    frame False {
                      n133 = Wait Until Next ms Multiple(millisecond multiple=u32 0) -> ()  [unwired: 1 out]
                    }
                    frame True {
                      n134 = Increment(x=w307) -> (x+1=w306:i32)
                      n135 = Enqueue Element(queue=w310, element=w308, error in (no error)=w311) -> (error out=w309:errorcluster)  [unwired: 1 in, 2 out]
                    }
                  }
                  n136 = control-ref of="Constellation Graph"() -> (w288:refnum<vi>)
                  n137 = call <vilib>:"MT Format Constellation.vi"("waveform"=w285, "constellation reference"=w288, "samples per symbol"=w287, "autoscale"="autoscale") -> ("constellation graph"=→"Constellation Graph":T10)  [unwired: 1 in, 10 out]
                  n138 = Equal?(x=1, y=w280) -> (x = y?=w284:bool)
                  n139 = Or(x=w283, y=w284) -> (x .or. y?=w282:bool)
                }
                n140 = while {
                  tunnel: TRUE -> [w279]
                  tunnel: [w279] -> w249
                  i -> [w277]
                  stop <- w276 stop-if-true
                  n141 = Equal?(x=0.0, y=w277) -> (x = y?=w276:bool)
                  "x = y?" <- w276
                  n142 = Wait Until Next ms Multiple(millisecond multiple="millisecond multiple 2") -> (millisecond timer value=→"millisecond timer value 4":u32)
                }
                "Boolean" <- w249
                n143 = Release Queue(queue=w268, error in (no error)=w267) -> (error out=w254:errorcluster)  [unwired: 3 out]
                n144 = call <instrlib>:"niUSRP Close Session.vi"("session handle"=w260, "error in (no error)"=w261) -> ("error out"=w253:errorcluster)  [unwired: 13 in]
                n145 = Merge Errors(w254, w253) -> (w252:errorcluster)
              }
              "error out 4" <- w224
              "Message Text 3" <- "Enter control signal (1,2 or 3)\n1. Power\n2. Trade Off\n3. Bandwidth"
            }
            frame #1 {
              n146 = Octal String To Number(4:w378) -> (0:w384:u32)  [unwired: 2 in, 1 out]
              n147 = Equal?(x=3, y=w384) -> (x = y?=w386:bool)
              n148 = Equal?(x=1, y=w384) -> (x = y?=w389:bool)
              n149 = Equal?(x=2, y=w384) -> (x = y?=w388:bool)
              n150 = Or(x=w389, y=w388) -> (x .or. y?=w387:bool)
              n151 = Or(x=w387, y=w386) -> (x .or. y?=w385:bool)
              n152 = while {
                tunnel: w385 -> [w394]
                tunnel: [w394] -> w380
                tunnel: w384 -> [w393]
                tunnel: [w393] -> w379
                i -> [w391]
                stop <- w390 stop-if-true
                n153 = Wait Until Next ms Multiple(millisecond multiple="millisecond multiple") -> (millisecond timer value=→"millisecond timer value 5":u32)
                n154 = Equal?(x=0.0, y=w391) -> (x = y?=w390:bool)
              }
              "Enter control signal (1,2 or 3)\n1. Power\n2. Trade Off\n3. Bandwidth 2" <- w378
            }
            frame #2 {
              n155 = case shown="False" w399 {
                tunnel: ["Not Done" "Switching Done"] -> w400
                tunnel: [_ w402] -> w397
                tunnel: w398 -> [_ w402]
                frame False {
                }
                frame True {
                }
              }
              "String" <- w400
            }
          }
          n156 = feedback #1() -> (w209:u32)  [unwired: 1 in]
          n157 = feedback-in #1(w210) -> ()
        }
      }
    }
  }
  n158 = feedback #2() -> (w1:i32)  [unwired: 1 in]
  n159 = feedback-in #2(w2) -> ()
  n160 = feedback #3() -> (w3:i32)  [unwired: 1 in]
  n161 = feedback-in #3(w4) -> ()
